vi "Argos 2.2 K1 Customized Edition.vi"(0 "PID 1 COM":refnum<visa-resource-name>="COM24", 1 "Setpoint\n START":bool, 2 "Write to File":bool, 3 "SP 1 input (°C)":dbl=10.0 min=0.0 max=1300.0, 4 "Intervall (s)":u32=1 max=600, 5 "Write/\nRead":bool=TRUE, 6 "Delay (ms)":u32=500 min=100 max=600000, 7 "Auto Tune":bool, 9 "Standby":bool, 11 "Reset\nSTOP":bool, 12 "ON":bool=TRUE caption="OFF", 13 "Get Values":bool, 15 "File Path":path) -> (8 "(°C)":dbl format="%#.3f", 14 "SP 1 is (°C)":dbl)   [LabVIEW 2013]
doc: "1. Verwendung\n\nDas Programm dient der Steuerung und Abfrage des Thermocontrollers I3252 und dem Auslesen von zwei VC 840 Messgeräten und einem Druckmessgerät Pfeiffer Single Gauge. \nDie Messgeräte werden Standardmäßig ausgelesen und erst nach Betätigung des Schalters \"Write to File\" in einer Textdatei abgespeichert. Das Eingabefeld \"Intervall\" legt den Abstand der Messpunkte fest.\nDer Setpoint für den Thermocontroller wird erst nach Betätigung des Tasters \"Setpoint START\" übernommen und angesteuert. Er wird ind den EEPROM des Gerätes geschrieben. Die Regelung kann mit Hilfe des Schalters \"Standby\" unterbrochen werden. Durch den Taster \"Reset STOPP\" kann der Setpoint aus dem EEPROM gelöscht werden.\nDie Eingabeflächen \"Constant\" und \"Thickness\" dienen der Berechnung des spezifischen Widerstands.\nDie Eingabeflächen \"User\" und \"Sample\" werden in den Header der Textdatei übernommen.\nDer Indikator \"File Path\" zeigt den aktuellen Speicherort der Textdatei an. Dieser wird nach ausschalten des Schalters \"Write to File\" gelöscht. Bei erneuten Schreiben muss ein neuer Speicherort gewählt werden. Bei Wahl desselben Speicherorts werden sämtliche bereits gespeicherte Daten gelöscht.\n\n\n2. Erläuterungen zum Blockdiagramm\n2.1 äußere Sequenz\nDie äußerte Sequenz besteht aus fünf Frames. Der erste dient der Initialisierung der Ports. Der zweite dient als Verzögerung um dem Programm genug Zeit zu geben die Ports zu öffnen. Jedoch senden die beiden VC 840 bereits Informationen an den Computer die in einem Puffer zwischengespeichert werden. Im dritten Frame wird dieser Puffer geleert. Somit kommt es zu keinem Framing Error. Desweiteren wird in diesem Frame die Startzeit der Messungen genommen. Im vierten Frame wird die eigentliche Messung und Verarbeitung der Daten durchgeführt. Die while-Schleife wird nur durch Auftreten eines Fehlers oder durch Betätigung des Stopbuttons auf dem Front Panel in der oberen linken Ecke unterbrochen. Im fünften und letzten Frame werden die Ports wieder geschlossen und beim Auftreten eines Fehlers wird das Programm automatisch gestoppt. Falls kein Fehler auftritt wird die Sequenz von vorne abgearbeitet.\n\n2.2 while-Schleife und innere Sequenz\n2.2.1 \"Event Structure\"\n2.2.1.1 Allgemein\nDer erste Frame beinhaltet ein \"Event Structure\". Dieser reagiert auf insgesamt elf verschiedene Ereignisse. Falls keines dieser Ereignisse auftreten sollte, warte die Struktur eine Millisekunde bevor die \"Event Structure\" verlassen wird. Die übrigen Ereignisse treten ein, wenn der entsprechende Kontroller eine Werteänderung erfährt.\n\n2.2.1.2 Event: Setpoint\nDieser Case besteht von außen nach innen aus einer Stacked Sequence, einer for-Loop und einer Flat Sequence die wiederum zwei \"Case Structures\" enthält. Als erstes wird bei dem Schalter \"Setpoint START\" der Blinkmodus aktiviert und bei dem Schalter \"Read Temperature\" deaktiviert. Danach folgt das eigentliche setzen des Temperatursollwerts. In der ersten Iteration wird dem Controller I3252 ein Schreibbefehl gesendet. Theoretisch kann der Setpoint in den RAM oder in den EEPROM geschrieben werden. Diese Auswahl erfolgt mit Hilfe des Schalters \"RAM\". Da das Schreiben in den RAM -Speicher aber aus diversen Gründen nicht erwünscht ist, wurde es nicht implementiert. Eine nachträgliche Implementierung ist aber leicht möglich, in dem die untere String-Konstante \"*P012\" durch \"*W012\" ersetzt wird. An diesem Befehl wird eine fünfstellige Hexadezimalzahl angehängt, die den Sollwert wiedergibt. Der Sollwert wird vorher mit zehn multipliziert, da das Komma standardmäßig nach der ersten Ziffer festgesetzt wurde (Bsp.: 800 wird gesendet um 80 einzustellen). Dieser Befehlsstrang wird an das Gerät mittels des SubVIs \"Comm_Interface\", auf welches später noch näher eingegangen wird, weitergegeben. Der durch das Gerät zurückgegebene String wird nicht verarbeitet.\nDie zweite Iteration dient dem Auslesen des eingestellten Sollwertes. Wahlweise kann der RAM- oder der EEPROM-Speicher ausgelesen werden. Die eigentliche Verarbeitung des Ausgabestrings erfolgt durch das SubVI \"Edit Setpoint\".\nDie Implementierung zur Einstellung des zweiten Setpoints erfolgt durch kopieren der ersten beiden Fälle und ersetzen der \"1\" im Befehf durch eine \"2\" (Bsp.: \"*P012\" zu \"*P022\"). Es darf aber nicht vergessen werden, dass dann ebenfalls die Anzahl der Iterationen angepasst werden muss.\nAls letztes wird der Blinkmodus des Schalters \"Setpoint START\" wieder deaktiviert.\n\n2.2.1.3 Event: Standby\nDieses Ereignis aktiviert bzw. deaktiviert als erstes den Blinckmodus des entsprechenden Schalters und sendet danach den Befehl zum aktivieren (\"*D03\") oder zum deaktivieren (\"*E03\") des Standbymodus an den Thermocontroller.\n\n2.2.1.4 Event: Set Command \nDer in das Feld \"Command shall be\" eingegebene Befehl wird an den Thermocontroller übermittlet. Die korrekte Form des Befehls ist im \"Communication Manuel\" nachzuschlagen. Das \"*\"-Zeichen wurde allerdings schon implementiert und muss somit nicht mit eingegeben werden.\n\n2.2.1.5 Event: Reset\nIn der ersten Iteration wird der Reset-Befehl an den Thermocontroller gesendet. In Folge wird der gesamte EEPROM-Speicher gelöscht. Deshalb wird in der zweiten Iteration der Setpoint aktualisiert. Dieser Befehl hat keinen Einfluss auf den RAM-Speicher. Die anschließende Wartezeit ist auf vier Sekunden festgesetzt und wurde empirisch ermittelt. Diese Zeit benötigt das Gerät um den Reset durchzuführen und für die Kommunikation wieder zur Verfügung zu stehen.\n\n2.2.1.6 Event: Auto Tune\nEs ist festgeschrieben, dass der Setpoint für die \"Auto Tune\"-Funktion wenigstens 20°C über der aktuellen Temperatur liegt. Deshalb wird zunächst der aktuelle Temperaturwert ausgelesen. Im zweiten Schritt werden zu diesem Wert zwanzig addiert und der Setpoint wird in den RAM-Speicher geschrieben. Das Schreiben in diesen Speicher ist nötig, da die \"Auto Tune\"-Funktion\" erst nach einem Reset startet. Im dritten Schritt wird der eigentliche Befehl für den \"Auto Tune\" gesendet (siehe dazu \"Communication Manuel\" S.27). Als vierte und letzte Iteration der for-Schleife folgt der bereits erwähnte Reset-Befehl. Der Temperatursollwert, der im RAM-Speicher eingetragen ist, muss zum Schluss wieder auf 0°C gesetzt werden. Die Zeit für die Ausführung des \"Auto Tune\"-Befehls wurde empirisch ermittelt und 45 s festgesetzt.\n\n2.2.1.7 Event: Write LOW/HI\nDieses Ereignis setzt die am Analogausgang anliegende Spannung fest. Normalerweise beträgt dieser Spannungswert 0-10 V. Das angeschlossene Netzteil verträgt aber maximal nur 2,3 V. Aus diesem Grund wird der \"%HIGH\" auf 23 gesetzt. Somit beträgt die maximal anliegende Spannung nur noch 23% von der maximal möglichen, d.h 2,3V. Ein niedrigerer Wert ist jederzeit möglich, genauso wie ein höherer für den Parameter \"%LOW\". Diese werden zunächst nacheinander in den RAM-Speicher geschrieben und anschließend wieder ausgelesen.\n\n2.2.1.8 Event: Set PID\nDie Werte für den PID-Regler können sowohl mit Hilfe der \"Auto Tune\"-Funktion, als auch manuell eingestellt werden. Es wird wiederum zwischen dem Schreiben in den RAM- und dem EEPROM-Speicher unterschieden. Zunächst werden die Werte für \"P\", \"I\" und \"D\", in dieser Reihenfolge, gesetzt und danach die aktuellen Werte ausgelesen.\n\n2.2.1.9 Event: Get Values\nDieses Ereignis hat zur Folge, dass die Werte für \"P\", \"I\", \"D\", \"%LOW\", \"%HIGH\" und des Setpoints wahlweise aus dem RAM- oder EEPROM-Speicher gelesen werden. Die aktuellen Werte werden nicht nur in die entsprechenden Anzeigefelder übernommen, sondern auch in die entsprechenden Eingabefelder, mit Ausnahme des Temperatursollwerts. \n\n2.2.1.10 Event: RAM\nPrinzipiell kann zwischen dem Schreiben in den RAM- oder EEPROM-Speicher des Thermocontrollers gewählt werden. Die entsprechende Schalterposition auf dem Frontpanel zeigt den aktuell verwendeten Speicher an. Die Anzeigewerte werden bei jedem Umschalten aktualisiert und sind im entsprechenden Speicher eingetragen. Die Implementierung ist identisch mit der des Ereignisses \"Get Values\". Es gilt zu beachten, dass die Werte für \"%LOW\" und \"%HIGH\" nur in den RAM-Speicher geschrieben werden können und somit auch nur aus diesem ausgelesen werden können.\n\n2.2.1.11 Event: Set Gauge to Zero\nMit Hilfe der SubVIs \"Get Pressure\" und \"Offset Display\" werden die Werte für den alten und den neuen Offset und der durch den zweiten Drucksensor ermittelt Druck ermittelt. \n\n2.2.1.12 Event: Write to File\nSollte der Schalter \"Write to File\" aktiviert werden, d.h. Schalterposition oben, so wird zunächst durch das SubVI \"Header\" ein Header für die unter \"File Path\" definierte Datei angelegt. Alle Werte, die bereits in der entsprechenden Datei stehen, werden dabei gelöscht.\n\n2.2.2 \"Timed Structures\"\nIm dritten Frame der inneren Sequenz werden die Werte für Zeitpunkt, Temperatur, Spannung, Strom und Druck ermittelt. Damit die Werte zum gleichen Zeitpunkt aufgenommen werden, werden \"Timed Sequences\" eingesetzt. Mit dem entsprechenden Schalter auf dem Front Panel unter dem Tab \"Settings\" kann gewählt werden, ob das entsprechende Gerät ausgelesen werden soll oder nicht. Die einzelnen Sequenzen werden parallel abgearbeitet, womit die Prozesszeit von diesem Frame durch der zeitintensivsten Sequenz abhängt. Dies ist in aller Regel das Auslesen der Temperatur, da ein \"Delay\" von 500 ms oder größer benötigt wird, um den Controller ordentlich ansprechen zu können.\nDie Systemzeit wird durch das SubVI \"System Time in Seconds\" in Sekunden umgerechnet und der in dem Parameter \"Starttime\" gespeicherte Wert wird abgezogen. Somit werden die Sekunden seit dem Start des Programms gezählt.\n\n2.2.3 restlichen Frames\nIm zweiten Frame wird das Intervall zwischen den einzelnen Messwerten festgelegt. Dabei wird der Wert des Parameters \"Delay\" abgezogen. Dieser Wert beträgt im Normalfall 500 ms und ist somit nicht vernachlääsigbar.\nDer Vierte Frame beinhaltet die Umrechnung des Temperatur-Strings in einen Temperaturwert durch das SubVI \"Edit Tmperature\", die Berechnung des spezifischen Widerstands durch das SubVI \"Resistivity Calculation\" und die Überprüfung des Druckwerts. Auch werden die neu gewonnen Werte in das entsprechende Shift-Register übernommen. Falls der Druckwert einen in dem Parameter \"Pressure Limit (mbar)\" festgelegten Grenzwert überschreiten sollte, wird der Thermocontroller automatisch in den Standby-Modus versetzt. Des Weiteren wird der Schalter \"Standby\" solange gesperrt, wie der Druck oberhalb des Grenzwertes liegt. Wenn der Druck wieder unter den Grenzwert gesunken ist, wird der Standby-Befehl nicht automatisch aufgehoben, sondern muss vom Benutzer durch Betätigung des entsprechenden Schalters gegeben werden.\nIm fünften Frame werden die Diagramme erstellt. Dabei wird jedes Mal von neuem das gesamte Shift-Register als Graph dargestellt. Weiterhin werden die Messwerte in ein 1D-Array geschrieben.\nDer sechste und letzte Frame beinhaltet den eigentlich Schreibvorgang der Messwerte in eine Textdatei und die Überprüfung ob ein Fehler vorliegt.\n\n2.3 SubVIs\n2.3.1 Allgemein\nDie SubVIs für die Messgeräte VC840 und das Druckmessgerät wurden aus anderen Quellen übernommen. \n\n2.3.2 \"Header\"\nIn den Header wird zunächst das aktuelle Datum und die aktuelle Zeit übernommen. Die ausgewählte Datei wird dabei überschrieben. Danach wird der Name des Benutzers und der Probe übernommen. Zum Schluss werden die Einheiten in einer Reihe, durch einen Tabulator getrennt, in den Header geschrieben.\n\n2.3.3 \"I3252 Comm Interface\"\nDieses VI stellt die Kommunikation mit dem Thermocontroller her und gibt den Ausgabe-String zurück.\n\n2.3.4 \"I3252 Edit Setpoint\"\nIm Ausgabe-String vom Thermocontroller ist an der vierten Stelle die Stelle des Dezimalpunktes verschlüsselt. Dieses Hexadezimalzahl wird herausgefiltert und an ein \"ENUM Controller\" übergeben. Dieser weist der Hexadezimalzahl eine Nummer zu, mit welcher ein Wert aus einem Array entnommen wird. Dieser Wert dient als Quotient. Der tatsächliche Wert kann somit errechnet werden.\n\n2.3.5 \"I3252 Edit Temperature\"\nDer Temperatur-String, der vom Thermocontroller zurückgegeben wird, wird in eine Dezimalzahl umgewandelt. Manchmal kommt es aus zu Dropouts, die durch dieses Programm herausgefiltert werden. Der letzte Wert wird dabei in einer \"Feedback Node\" gehalten unter der Annahme, dass sich der Temperaturwert nicht sprunghaft ändert.\n\n2.3.6 \"Resistivity Calculation\"\nDer spezifische Widerstand wird nach folgender Formel ausgerechnet. Dabei entspricht t der Dicke der Probe und C ist eine Konstante.\nrho=C*pi*t*U/(ln( 2)*I)\n\n2.3.7 \"System Time in Seconds\"\nZunächst wird die aktuelle Systemzeit ausgelesen. Danach wird diese in Stunden, Minuten und Sekunden aufgeteilt, alles in Sekunden umgerechnet und letztendlich addiert."
uses:
  <vilib>/Platform/TimedLoop/XDataNode/timing_clust.ctl
  <vilib>/Platform/TimedLoop/XDataNode/nitl_modes.ctl
  <vilib>/Platform/TimedLoop/XDataNode/wakeup.ctl
  <vilib>/Instr/_visa.llb/VISA Configure Serial Port (Instr).vi
  <vilib>/Platform/TimedLoop/scheduler/LVUserAPI/_suppVIs/Create_1kHz_TSource.vi
  <vilib>/Utility/file.llb/Write To Spreadsheet File (DBL).vi
  <vilib>/Platform/TimedLoop/XDataNode/XDataNode.xnode
  <vilib>/Platform/TimedLoop/XDataNode/XDNodeRunTimeDep.lvlib
  Argos2.0/Dependencies/Pfeiffer TPG261+262 Single+Dual Gauge/Dual Gauge.lvlib
panel:
  out "appended array":dbl[](array[numeric])
  in  "Tab Control":T1(tab)
  out "SP 2 is (°C)":dbl
  in  "SP 2 input (°C)":dbl=10.0 min=0.0 max=1300.0
  in  "Standby\n2":bool
  in  "Setpoint\n START\n2":bool
  out "Pirani (VVP1 Scroll)":cluster{dbl[], dbl[]}[](graph)
  in  "Sample":string
  in  "User":string
  out "current time (s)":dbl
  out "data logger intervall (s)":dbl
  out "loop time (s)":dbl
  in  "stop":bool
  out "CMR275 Baratron":cluster{dbl[], dbl[]}(graph)
  out "Pressure Baratron 2":dbl format="%#_4e"
  out "Pressure FullRange 2":dbl format="%#_3e"
  out "Pressure Pirani 2":dbl format="%#_3e"
  in  "Reset\nSTOP 2":bool
  out "TEMPERATURE":cluster{dbl[], dbl[]}[](graph)
  out "(°C) 2":dbl format="%#.3f"
  out "Pressure OpenPort":cluster{dbl[], dbl[]}(graph)
  out "Pressure OpenPort2":dbl caption="current"
  out "% HIGH Istwert 2":u32
  out "% LOW Istwert 2":u32
  in  "% High Sollwert 2":u32=23 max=24
  in  "% LOW Sollwert 2":u32 max=25
  in  "RAM 2":bool=TRUE caption="EEPROM"
  out "D (Rate) IstWert 2":u32
  out "I ( Reset1) Istwert 2":u32
  out "P (PB1) Istwert 2":u32 caption="actual value"
  in  "D (Rate) Sollwert 2":u32 max=3999
  in  "I ( Reset1) Sollwert 2":u32 max=3999
  in  "P (PB1) Sollwert 2":u32 caption="set value" max=9999
  in  "ON 2":bool=TRUE caption="OFF"
  in  "PID 2 COM":refnum<visa-resource-name>="COM25"
  in  "Delay (ms) 2":u32=500 min=100 max=600000
  in  "Write/\nRead \n\n2":bool=TRUE
  out "status 2":bool caption="Status"
  out "code 2":i32 caption="Code"
  out "code":i32 caption="Code"
  out "status":bool caption="Status"
  in  "Set Gauge to Zero":bool
  out "Status Gauge 1#2":i32(ring) items=["data OK", "underrange", "overrange", "sensor error", "sensor off", "no sensor", "ID error"]
  out "Pressure Gauge 1#2":dbl format="%.3e"
  out "Pressure Gauge 1#1":dbl format="%.3e"
  out "Status Gauge 1#1":i32(ring) items=["data OK", "underrange", "overrange", "sensor error", "sensor off", "no sensor", "ID error"]
  in  "TPG 1 COM":refnum<visa-resource-name>="COM23"
  in  "Pressure Limit (mbar)":dbl=1.0 min=0.0 max=1100.0
  out "Current Offset (mbar)":dbl
  in  "ON (TPG 2)":bool=TRUE caption="OFF"
  in  "ON (TPG 1)":bool=TRUE caption="OFF"
  in  "ON":bool caption="OFF"
  in  "VC 840 2":refnum<visa-resource-name>="COM8"
  out "Reading 2":dbl format="%_4f"
  out "Mode 2":enum16{"?", "Diode", "Beep", "DC", "AC"}(ring)
  out "Unit 2":string
  in  "VC 840 1":refnum<visa-resource-name>="COM1"
  out "Reading 1":dbl format="%_4f"
  out "Mode 1":enum16{"?", "Diode", "Beep", "DC", "AC"}(ring)
  out "Unit 1":string
  out "Status 1":T2
  out "Status 2":T2
  in  "ON":bool caption="OFF"
  out "% HIGH Istwert":u32
  out "% LOW Istwert":u32
  in  "% High Sollwert":u32=23 max=24
  in  "% LOW Sollwert":u32 max=25
  in  "RAM":bool=TRUE caption="EEPROM"
  out "D (Rate) IstWert":u32
  out "I ( Reset1) Istwert":u32
  out "P (PB1) Istwert":u32 caption="actual value"
  in  "D (Rate) Sollwert":u32 max=3999
  in  "I ( Reset1) Sollwert":u32 max=3999
  in  "P (PB1) Sollwert":u32 caption="set value" max=9999
  in  "Set Command":bool
  in  "Set PID":bool
  in  "Write LOW/HI":bool
  out "Command output":string
  in  "Command input":string
  in  "TPG 2 COM":refnum<visa-resource-name>="COM22"
  out "Pressure Gauge 2#2":dbl format="%.3e"
  out "Pressure Gauge 2#1":dbl format="%.3e"
  out "Status Gauge 2#2":i32(ring) items=["data OK", "underrange", "overrange", "sensor error", "sensor off", "no sensor", "ID error"]
  out "Status Gauge 2#1":i32(ring) items=["data OK", "underrange", "overrange", "sensor error", "sensor off", "no sensor", "ID error"]
  out "Command output 2":string
  in  "Command input 2":string
  in  "Set Command\n\n 2":bool
  in  "Auto Tune 2":bool
  in  "Set PID 2":bool
  in  "Write LOW/HI 2":bool
  in  "Get Values 2":bool
  out "Current":cluster{dbl[], dbl[]}(graph)
  out "Voltage":cluster{dbl[], dbl[]}(graph)
  out "Voltage (V)":dbl format="%.4e"
  out "Current (A)":dbl format="%.4e"
  out "Resistivity":cluster{dbl[], dbl[]}(graph)
  out "Resistivity (Ohm*cm)":dbl format="%.3e"
  in  "4PP constant":dbl min=0.0 max=5.0
  in  "Thickness (nm)":dbl min=0.0
  # "PID Side A"
  # "PID Side B"
  # "set \nvalue"
  # "actual \nvalue"
  # "Set \nValue\n2"
  # "Actual \nvalue 2"
  # "T (°C)"
  # "T (°C)"
  # "mbar"
  # "mbar"
  # "mbar"
  # "mbar"
  # "Pressure Measurement \n(Pfeiffer TPG261)"
  # "PID Controller (Omega Newport i3252)"
  # "PID Controller 2 (Omega Newport i3252)"
  # "P"
  # "I"
  # "D"
  # "% Low"
  # "% High"
  # "Multimeter\n#1 (VC 840)"
  # "Multimeter\n#2 (VC 840)"
  # "P"
  # "I"
  # "D"
  # "% Low"
  # "% High"
  # "Authors:  Daniel Schuster (sir-dan@web.de)\n                 Steffen Cornelius (s.cornelius@hzdr.de)\n                 Nico Spahn (x)\n\n                 premade SubVIs for readout of Pfeiffer gauge and VC840 Multimeters were used\n                 SubVI \"I3252_Comm_Interface\" is based on a modified Labview example\n\nRelease:  v1.0    \n\nVersion History:\n\nv1.1  -    28.06.2011\n             - Format des Files geändert von %.3f auf %g\n             - maximale Eingabewerte für PID begrenzt\nv1.2  -    12.07.2011\n             - Anzeige p,rho, U, V auf Scientific geändert\n             - y-Achse p,rho auf Log geändert\n             - numerische Zeitanzeige hinzugefügt\n             - 4PP Constant: pi/ln(2)=4,532 set as the default value\nv1.3  -    25.07.2011\n             - Zeitvariable auf EXT geändert, um Sprünge in Diagrammen loszuwerden\nv1.4  -   27.07.2011\n             - ALLE Variablen auf DBL zurückgesetzt wegen Formatierungsproblem im File\n             - Zeitberechnung neu gemacht (Tick count differenzen) -> Zeitsprünge korrigiert ?\n             - Delay/Intervall überarbeitet\nv1.5  -   05.12.2012\n                - Austausch der alten Pfeifer SubvIs durch neue -> nun alle 4 Kanäle des DualGauge\n                                                                                                         Controllers gleichzeitig auslesbar\n                - neue Pfeiffer SubVIs verwendet in Druckwertauslesung und Offset Berechnung des Baratron\n                  Druckes (COM5 Sensor1)\n                - Neuarragement des GUI -> FullRange und Baratron neben Temperatur auf Haupseite zu sehen\n                                                                   Pirani und OpenPort auf Meas.2 zu sehen\n                                                                   Diagnose Seite umfasst nun auch Widerstandsdiagramm\n                - Änderungen der Settingseite -> nun alle 4 Drucksensoren mit aktuellem Messwert und Gerätestatus\n                                                                           zu sehen\n                - The readout of the PID-Temperature Controller and the VC840 Multimeters was not modified\nv1.73  -  18.10.2013\n                - Layout Änderungen\nv.1.8   -  19.01.2014\n                - Änderung Layout Settings Tab\n                - Trennung der beiden TPG Dual Gauge Controls\n                -"
  # "Version 1.73    - last change 18.10.2013"
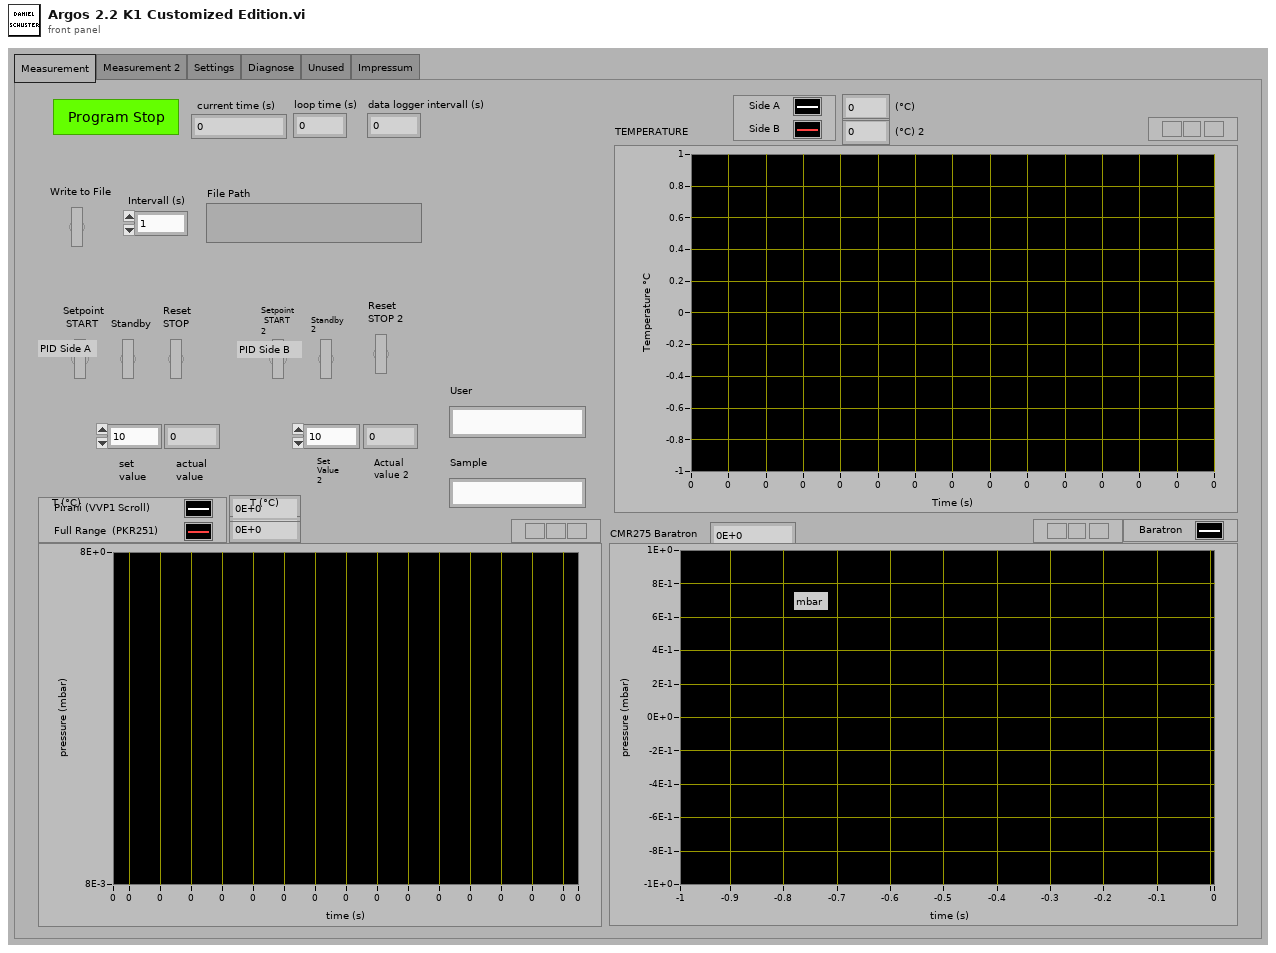
[diagram p1: front panel]
types:
  T1 = enum32{"Measurement", "Measurement 2", "Settings", "Diagnose", "Unused", "Impressum"}
  T2 = cluster{"Low Bat":bool, "Auto":bool, "Delta":bool, "Hold":bool, "RS232":bool}
  T3 = typedef "XDNodeRunTimeDep.lvlib/timing_clust.ctl" = cluster{"Expected End [f-1]":u64, "Actual End [f-1]":u64, "Finished Late? [f-1]":bool, "Expected End [i-1]":u64, "Actual End [i-1]":u64, "Finished Late? [i-1]":bool, "Expected Start [i]":u64, "Actual Start [i]":u64, "Expected Start [f]":u64, "Actual Start [f]":u64, "Source Name":string, "Structure Name":string, "Period":i64, "Deadline":i64, "Offset":i64, "Start":i64, "Priority":i32, "Timeout":i32, "Mode":T4, "Wakeup Reason":T5, "Error":errorcluster, "Source Type":string, "Secondary Source Type":string, "Global End Time":u64, "Global Start Time":u64, "Frame Duration":u64, "Iteration Duration":u64, "Assigned CPU":i32, "I/O Scan Engine Mode":u32}
  T4 = typedef "XDNodeRunTimeDep.lvlib/nitl_modes.ctl" = enum32{"No Change", "Process missed periods, maintain original phase", "Discard missed periods, maintain original phase", "Process missed periods, ignore original phase", "Discard missed periods, ignore original phase"}
  T5 = typedef "XDNodeRunTimeDep.lvlib/wakeup.ctl" = enum32{"Normal", "Aborted", "Asynchronous wakeup", "Timing source error", "Timed loop error", "Timeout"}
  T6 = enum8{"Enabled", "Disabled", "Disabled and Grayed Out"}
  T7 = cluster{"VISA resource name out":refnum<visa-resource-name>, "error out":errorcluster, "Delay (ms)":u32, "Write/\nRead":bool}
  T8 = cluster{"VISA resource name out":refnum<visa-resource-name>, "error out":errorcluster, "Delay (ms) 2":u32, "Write/\nRead \n\n2":bool}
  T9 = cluster{"TPG 2 COM":refnum<visa-resource-name>, "error out":errorcluster}
  T10 = cluster{"COM out":refnum<visa-resource-name>, "Cluster (Ausgang)":errorcluster}
  T11 = cluster{"Pressure Gauge#1":dbl, "Pressure Gauge#2":dbl}
  T12 = cluster{"TPG 1 COM":refnum<visa-resource-name>, "error out":errorcluster}
  T13 = cluster{"COM out":refnum<visa-resource-name>, "error out":errorcluster, "COM out":refnum<visa-resource-name>, "error out":errorcluster}
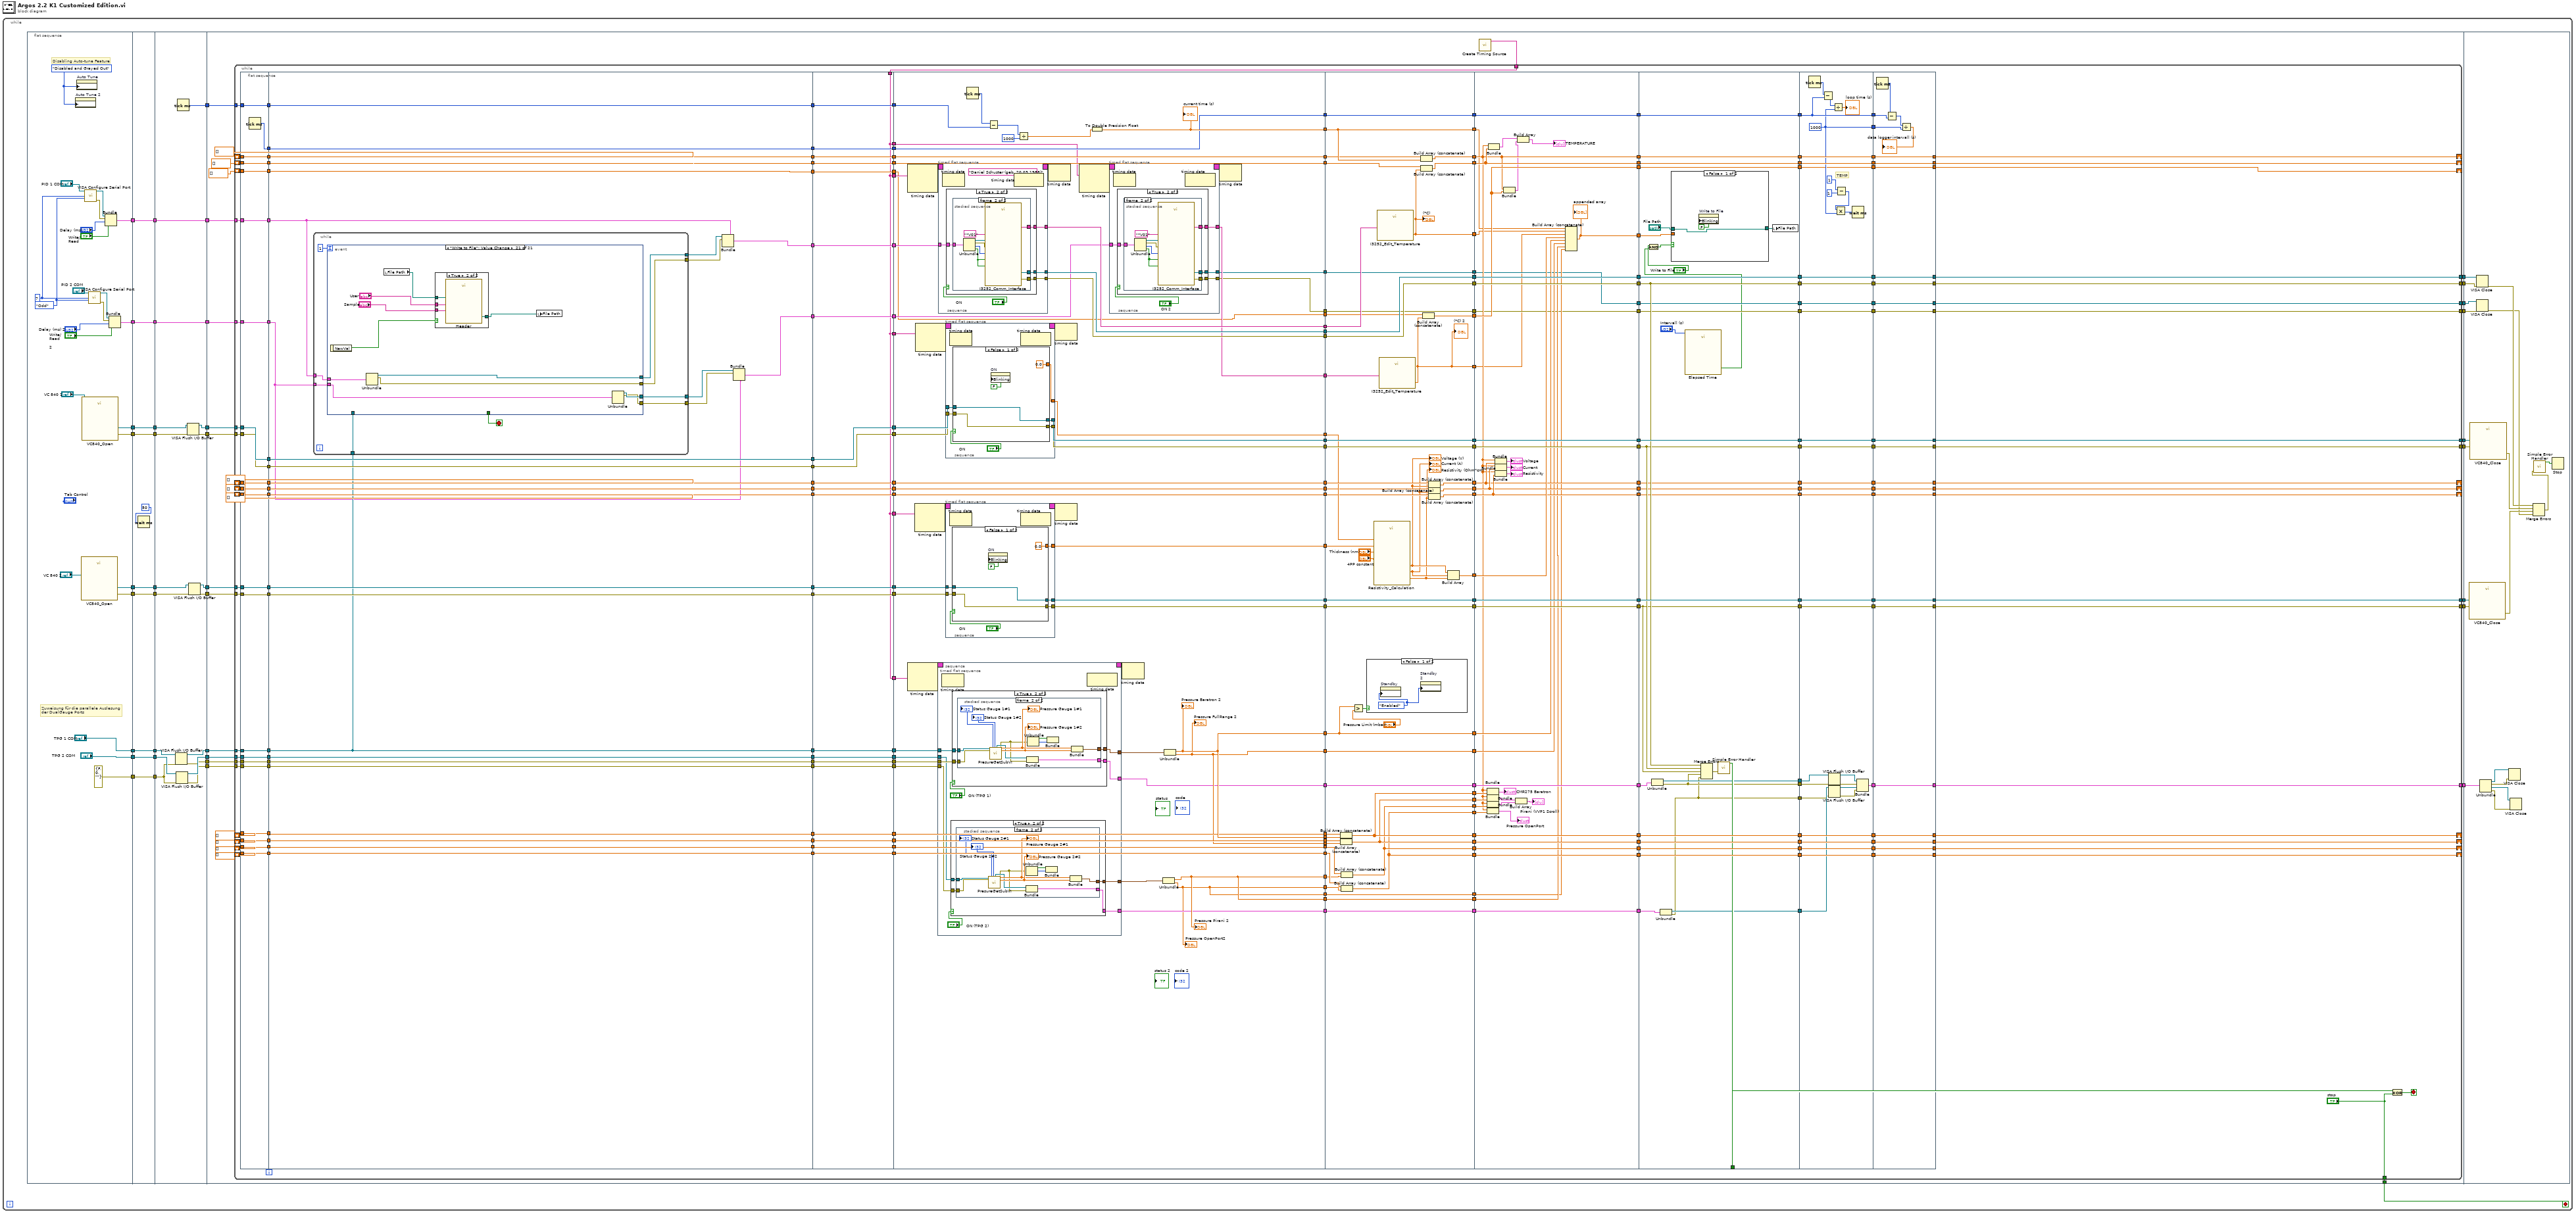
[diagram p0: block diagram]
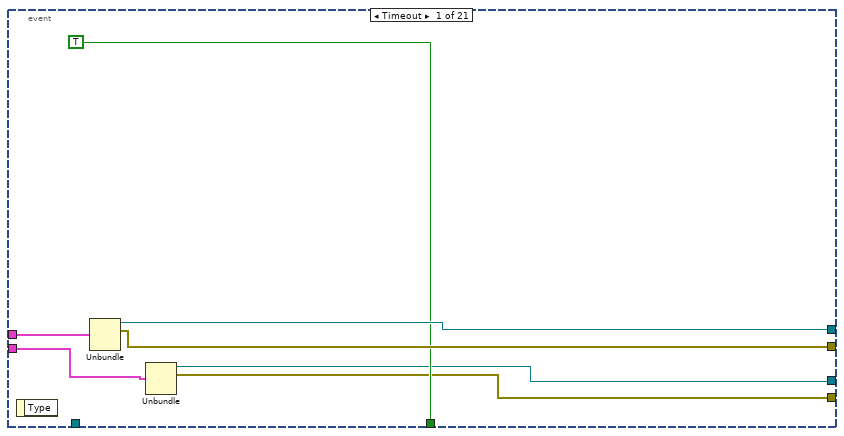
[diagram p2: hidden frame]
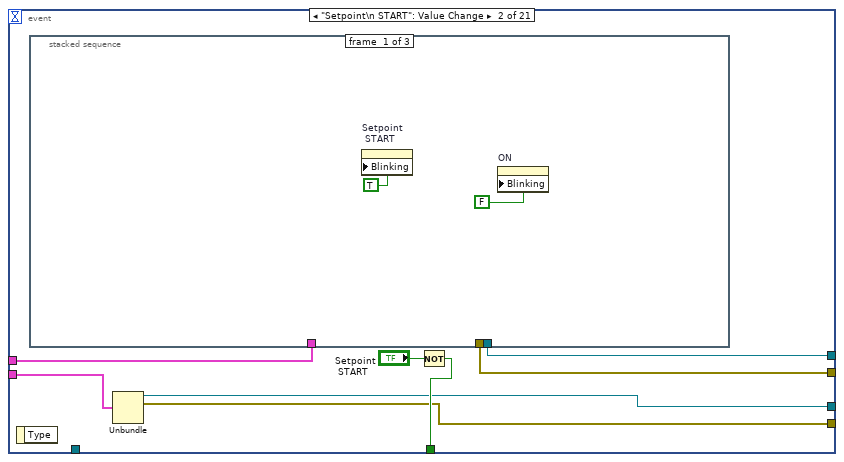
[diagram p3: hidden frame]
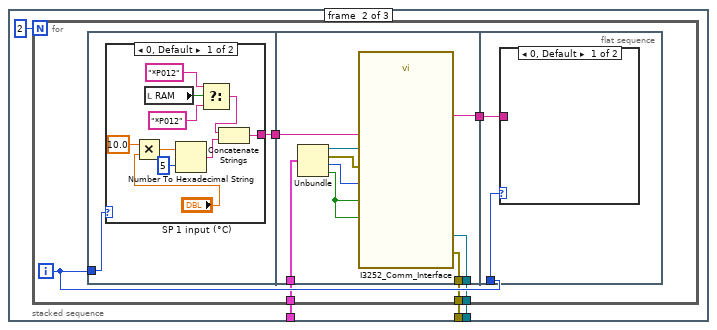
[diagram p4: hidden frame]
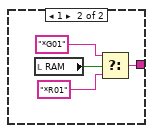
[diagram p5: hidden frame]
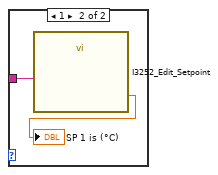
[diagram p6: hidden frame]
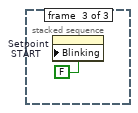
[diagram p7: hidden frame]
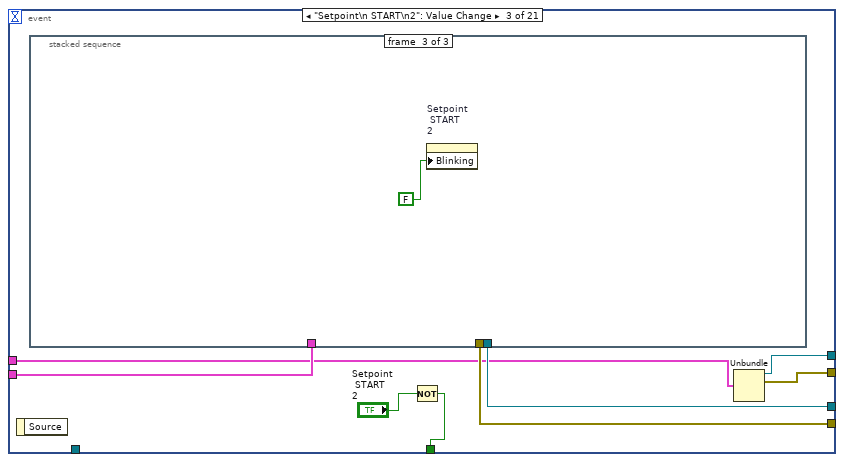
[diagram p8: hidden frame]
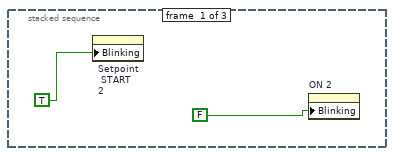
[diagram p9: hidden frame]
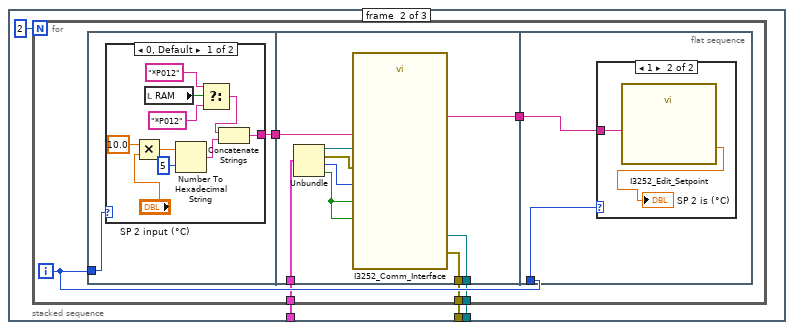
[diagram p10: hidden frame]
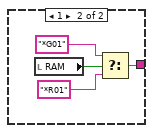
[diagram p11: hidden frame]
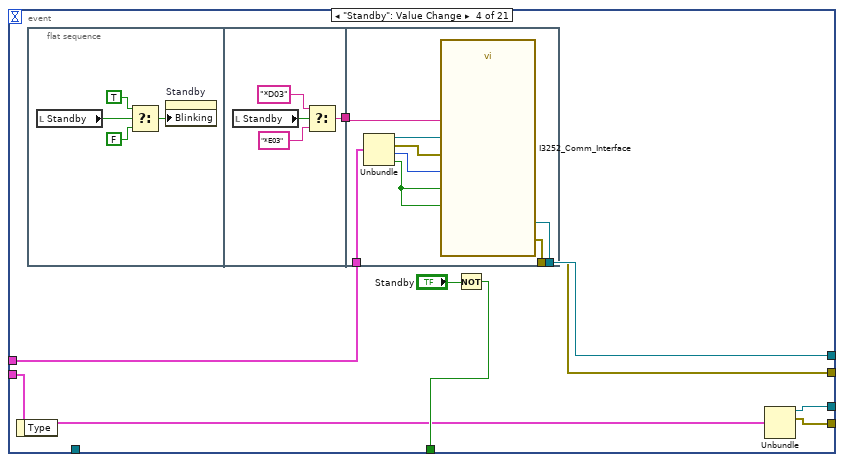
[diagram p13: hidden frame]
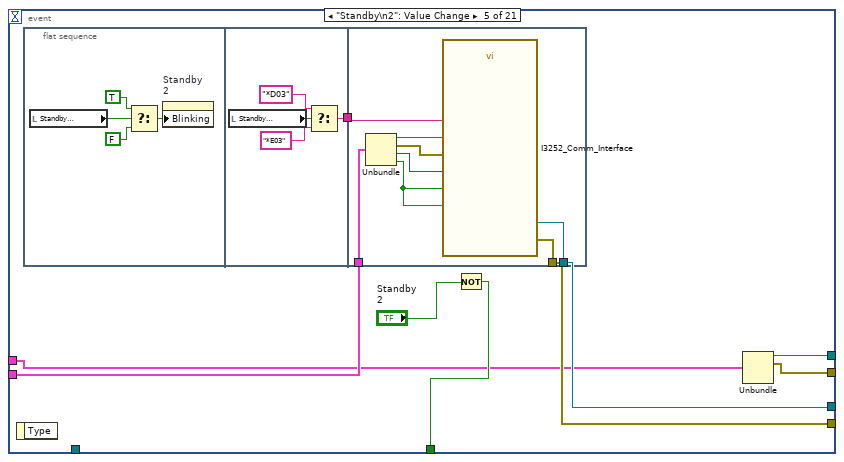
[diagram p14: hidden frame]
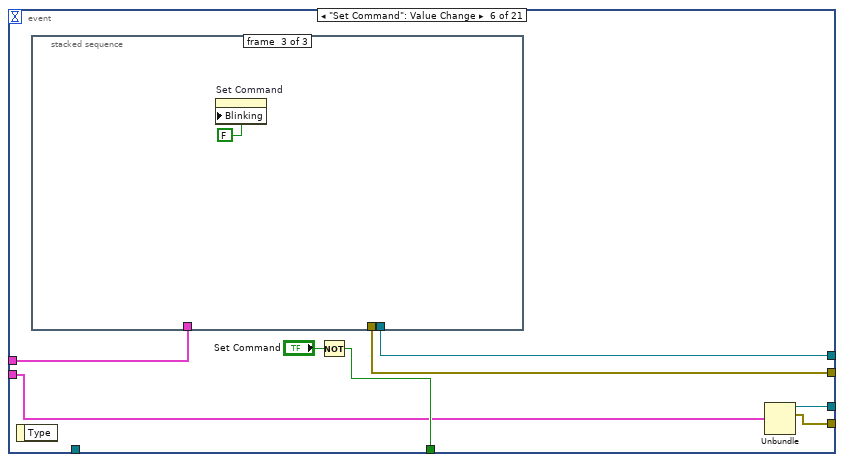
[diagram p15: hidden frame]
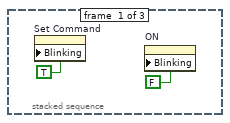
[diagram p16: hidden frame]
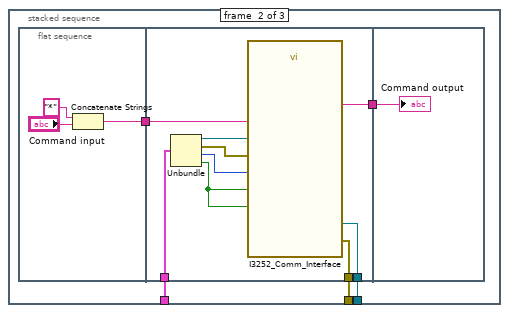
[diagram p17: hidden frame]
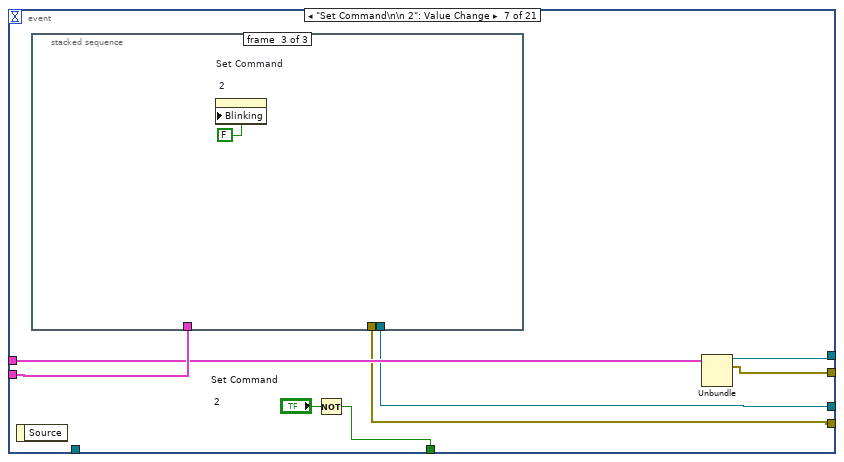
[diagram p18: hidden frame]
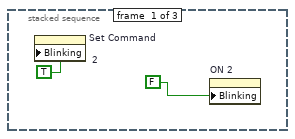
[diagram p19: hidden frame]
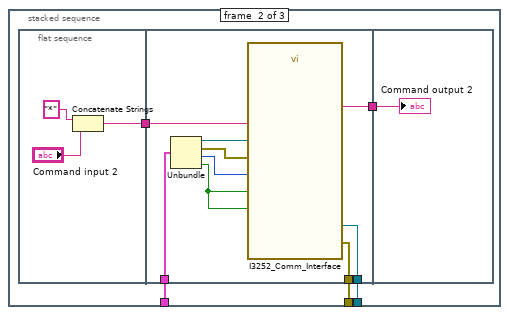
[diagram p20: hidden frame]
diagram:
  n1 = while {
    stop <- w11 stop-if-true
    n2 = flat-sequence {
      tunnel: [w62] -> w39
      tunnel: [w63] -> w38
      tunnel: [w54] -> w37
      tunnel: [w61] -> w36
      tunnel: [w60] -> w35
      tunnel: ["TPG 1 COM"] -> w34
      tunnel: ["TPG 2 COM"] -> w33
      tunnel: [errorcluster {"status"=FALSE, "code"=0, "source"=""} ("Fehler (Eingang)")] -> w8
      tunnel: [w43] -> w3
      tunnel: w39 -> [w73]
      tunnel: [w73] -> w32
      tunnel: w38 -> [w72]
      tunnel: [w72] -> w31
      tunnel: w37 -> [w71]
      tunnel: [w71] -> w30
      tunnel: w36 -> [w70]
      tunnel: [w70] -> w29
      tunnel: w35 -> [w69]
      tunnel: [w69] -> w28
      tunnel: [w67] -> w27
      tunnel: w34 -> [w67]
      tunnel: [w66] -> w26
      tunnel: w33 -> [w66]
      tunnel: [w65] -> w9
      tunnel: w8 -> [w65]
      tunnel: [w64] -> w4
      tunnel: w3 -> [w64]
      tunnel: w32 -> [w85]
      tunnel: [w84] -> w25
      tunnel: w31 -> [w86]
      tunnel: [w83] -> w24
      tunnel: w30 -> [w91]
      tunnel: [w91] -> w23
      tunnel: w29 -> [w88]
      tunnel: [w89] -> w22
      tunnel: w28 -> [w87]
      tunnel: [w90] -> w21
      tunnel: [w82] -> w20
      tunnel: [w80] -> w19
      tunnel: w27 -> [w81]
      tunnel: [w79] -> w18
      tunnel: w26 -> [w78]
      tunnel: w9 -> [w77]
      tunnel: [w76] -> w7
      tunnel: [w75] -> w6
      tunnel: [w74] -> w5
      tunnel: w4 -> [w74]
      tunnel: w25 -> [w123]
      tunnel: w24 -> [w122]
      tunnel: w23 -> [w121]
      tunnel: w22 -> [w119]
      tunnel: w21 -> [w118]
      tunnel: [w117] -> w17
      tunnel: [w116] -> w16
      tunnel: [w115] -> w15
      tunnel: [w114] -> w14
      tunnel: [w113] -> w13
      tunnel: [w112] -> w12
      tunnel: w20 -> [w106]
      tunnel: w19 -> [w105]
      tunnel: w18 -> [w104]
      tunnel: [w99] -> w11
      tunnel: [w98] -> w10
      tunnel: w7 -> [w97]
      tunnel: w6 -> [w96]
      tunnel: w5 -> [w95]
      tunnel: [w94] -> w2
      tunnel: [w93] -> w1
      tunnel: w17 -> [w1960]
      tunnel: w16 -> [w1959]
      tunnel: w15 -> [w1962]
      tunnel: w14 -> [w1961]
      tunnel: w13 -> [w1964]
      tunnel: w12 -> [w1963]
      tunnel: w10 -> [w1957]
      tunnel: w2 -> [w1952]
      tunnel: w1 -> [w1951]
      frame #0 {
        w41 = u16 7 ("data bits (8)")
        w40 = enum16{"None", "Odd", "Even", "Mark", "Space"}."Odd" ("parity (0:none)")
        w42 = T6."Disabled and Grayed Out" ("Disabled")
        # "Disabling Auto-tune Feature"
        # "Zuweisung für die parallele Auslesung\nder DualGauge Ports"
        n3 = property on="Auto Tune 2" class="Bool"("DisabledEnum"=w42) -> ()  [unwired: 2 in, 2 out]
        n4 = property on="Auto Tune" class="Bool"("DisabledEnum"=w42) -> ()  [unwired: 2 in, 2 out]
        n5 = call "VC840_Open.vi"("VISA resource name"="VC 840 2") -> ("error out"=w60:errorcluster, "VISA resource name out"=w61:refnum<visa-resource-name>)  [unwired: 1 in, 8 out]
        n6 = call "VC840_Open.vi"("VISA resource name"="VC 840 1") -> ("error out"=w63:errorcluster, "VISA resource name out"=w62:refnum<visa-resource-name>)  [unwired: 1 in, 8 out]
        n7 = call-poly "VISA Configure Serial Port"("VISA resource name"="PID 1 COM", "data bits (8)"=w41, "parity (0:none)"=w40) -> ("VISA resource name out"=w58:refnum<visa-resource-name>, "error out"=w59:errorcluster)  [unwired: 6 in, 5 out]
        n8 = call-poly "VISA Configure Serial Port"("VISA resource name"="PID 2 COM", "data bits (8)"=w41, "parity (0:none)"=w40) -> ("VISA resource name out"=w47:refnum<visa-resource-name>, "error out"=w48:errorcluster)  [unwired: 6 in, 5 out]
        n9 = Bundle("VISA resource name out"=w58, "error out"=w59, "Delay (ms)"="Delay (ms)", "Write/\nRead"="Write/\nRead") -> (w54:T7)  [unwired: 1 in]
        n10 = Bundle("VISA resource name out"=w47, "error out"=w48, "Delay (ms) 2"="Delay (ms) 2", "Write/\nRead \n\n2"="Write/\nRead \n\n2") -> (w43:T8)  [unwired: 1 in]
      }
      frame #1 {
        n11 = Wait (ms)(milliseconds to wait=u32 50) -> ()  [unwired: 1 out]
      }
      frame #2 {
        n12 = VISA Flush I/O Buffer(VISA resource name=w81, error in (no error)=w77) -> (VISA resource name out=w80:refnum<visa-resource-name>, error out=w76:errorcluster)  [unwired: 1 in]
        n13 = VISA Flush I/O Buffer(VISA resource name=w78, error in (no error)=w77) -> (VISA resource name out=w79:refnum<visa-resource-name>, error out=w75:errorcluster)  [unwired: 1 in]
        n14 = Tick Count (ms)() -> (millisecond timer value=w82:u32)
        n15 = VISA Flush I/O Buffer(VISA resource name=w85, error in (no error)=w86) -> (VISA resource name out=w84:refnum<visa-resource-name>, error out=w83:errorcluster)  [unwired: 1 in]
        n16 = VISA Flush I/O Buffer(VISA resource name=w88, error in (no error)=w87) -> (VISA resource name out=w89:refnum<visa-resource-name>, error out=w90:errorcluster)  [unwired: 1 in]
      }
      frame #3 {
        n17 = call-poly <vilib>:"Create Timing Source.vi"() -> ("name (out)"=w120:string)  [unwired: 10 in, 1 out]
        n18 = while {
          tunnel: w123 -> [w371]
          tunnel: w122 -> [w370]
          tunnel: w121 -> [w369]
          tunnel: w120 -> [w362]
          tunnel: w119 -> [w355]
          tunnel: w118 -> [w354]
          tunnel: [w350] -> w117
          tunnel: [w349] -> w116
          tunnel: [w347] -> w115
          tunnel: [w345] -> w114
          tunnel: [w343] -> w113
          tunnel: [w341] -> w112
          shift-right: [w314] -> _
          shift-left: dbl[] [] -> [w319]
          shift-right: [w292] -> _
          shift-left: dbl[] [] -> [w327]
          shift-right: [w316] -> _
          shift-left: dbl[] [] -> [w323]
          shift-right: [w289] -> _
          shift-left: dbl[] [] -> [w326]
          shift-right: [w286] -> _
          shift-left: dbl[] [] -> [w325]
          tunnel: w106 -> [w280]
          tunnel: w105 -> [w236]
          tunnel: w104 -> [w232]
          shift-right: [w190] -> _
          shift-left: dbl[] [] -> [w220]
          shift-right: [w188] -> _
          shift-left: dbl[] [] -> [w218]
          shift-right: [w186] -> _
          shift-left: dbl[] [] -> [w216]
          shift-right: [w184] -> _
          shift-left: dbl[] [] -> [w214]
          tunnel: ["stop"] -> w99
          tunnel: [w178] -> w98
          tunnel: w97 -> [w173]
          tunnel: w96 -> [w171]
          tunnel: w95 -> [w151]
          shift-right: [w143] -> _
          shift-left: dbl[] [] -> [w141]
          tunnel: [w132] -> w94
          tunnel: [w126] -> w93
          stop <- w177 stop-if-true
          n19 = flat-sequence {
            tunnel: w280 -> [w383]
            tunnel: w319 -> [w384]
            tunnel: w323 -> [w385]
            tunnel: w325 -> [w386]
            tunnel: w326 -> [w387]
            tunnel: w327 -> [w388]
            tunnel: w354 -> [w389]
            tunnel: w355 -> [w390]
            tunnel: w369 -> [w391]
            tunnel: w370 -> [w392]
            tunnel: w371 -> [w393]
            tunnel: [w393] -> w279
            tunnel: [w392] -> w278
            tunnel: [w391] -> w277
            tunnel: [w390] -> w276
            tunnel: [w389] -> w275
            tunnel: [w388] -> w274
            tunnel: [w387] -> w273
            tunnel: [w386] -> w272
            tunnel: [w385] -> w271
            tunnel: [w384] -> w270
            tunnel: [w383] -> w269
            tunnel: [w382] -> w251
            tunnel: [w381] -> w237
            tunnel: w236 -> [w381]
            tunnel: [w380] -> w233
            tunnel: w232 -> [w380]
            tunnel: [w379] -> w221
            tunnel: w220 -> [w379]
            tunnel: [w378] -> w219
            tunnel: w218 -> [w378]
            tunnel: [w377] -> w217
            tunnel: w216 -> [w377]
            tunnel: [w376] -> w215
            tunnel: w214 -> [w376]
            tunnel: [w375] -> w174
            tunnel: w173 -> [w375]
            tunnel: [w374] -> w172
            tunnel: w171 -> [w374]
            tunnel: [w373] -> w152
            tunnel: w151 -> [w373]
            tunnel: [w372] -> w142
            tunnel: w141 -> [w372]
            tunnel: [w421] -> w368
            tunnel: [w420] -> w366
            tunnel: [w416] -> w364
            tunnel: [w415] -> w359
            tunnel: [w414] -> w357
            tunnel: [w413] -> w324
            tunnel: [w412] -> w320
            tunnel: [w411] -> w300
            tunnel: [w410] -> w297
            tunnel: [w409] -> w295
            tunnel: [w408] -> w281
            tunnel: w279 -> [w421]
            tunnel: w278 -> [w420]
            tunnel: w277 -> [w419]
            tunnel: w276 -> [w415]
            tunnel: w275 -> [w414]
            tunnel: w274 -> [w411]
            tunnel: w273 -> [w410]
            tunnel: w272 -> [w409]
            tunnel: w271 -> [w413]
            tunnel: w270 -> [w412]
            tunnel: w269 -> [w408]
            tunnel: [w407] -> w252
            tunnel: w251 -> [w407]
            tunnel: w237 -> [w405]
            tunnel: [w405] -> w234
            tunnel: w233 -> [w406]
            tunnel: [w406] -> w230
            tunnel: w221 -> [w404]
            tunnel: w219 -> [w403]
            tunnel: w217 -> [w402]
            tunnel: w215 -> [w401]
            tunnel: [w404] -> w213
            tunnel: [w403] -> w209
            tunnel: [w402] -> w206
            tunnel: [w401] -> w205
            tunnel: w174 -> [w400]
            tunnel: w172 -> [w399]
            tunnel: [w400] -> w169
            tunnel: [w399] -> w167
            tunnel: w152 -> [w395]
            tunnel: [w394] -> w149
            tunnel: w142 -> [w398]
            tunnel: [w398] -> w140
            tunnel: w368 -> [w1472]
            tunnel: [w1472] -> w367
            tunnel: w366 -> [w1471]
            tunnel: [w1471] -> w365
            tunnel: w364 -> [w1468]
            tunnel: [w1468] -> w363
            tunnel: w362 -> [w1450]
            tunnel: [w1450] -> w361
            tunnel: [w1450] -> w360
            tunnel: w359 -> [w1470]
            tunnel: [w1470] -> w358
            tunnel: w357 -> [w1469]
            tunnel: [w1469] -> w356
            tunnel: [w1450] -> w353
            tunnel: [w1450] -> w339
            tunnel: w324 -> [w1467]
            tunnel: [w1467] -> w322
            tunnel: w320 -> [w1466]
            tunnel: [w1466] -> w317
            tunnel: [w1465] -> w301
            tunnel: w300 -> [w1465]
            tunnel: [w1464] -> w298
            tunnel: w297 -> [w1464]
            tunnel: [w1463] -> w296
            tunnel: w295 -> [w1463]
            tunnel: [w1462] -> w282
            tunnel: w281 -> [w1462]
            tunnel: [w1461] -> w253
            tunnel: w252 -> [w1461]
            tunnel: [w1460] -> w235
            tunnel: w234 -> [w1460]
            tunnel: [w1459] -> w231
            tunnel: w230 -> [w1459]
            tunnel: w213 -> [w1458]
            tunnel: [w1458] -> w212
            tunnel: [w1457] -> w210
            tunnel: w209 -> [w1457]
            tunnel: [w1456] -> w208
            tunnel: w206 -> [w1456]
            tunnel: w205 -> [w1455]
            tunnel: [w1455] -> w204
            tunnel: [w1454] -> w170
            tunnel: w169 -> [w1454]
            tunnel: [w1453] -> w168
            tunnel: w167 -> [w1453]
            tunnel: [w1452] -> w150
            tunnel: w149 -> [w1452]
            tunnel: w140 -> [w1451]
            tunnel: [w1451] -> w139
            tunnel: [w1450] -> w125
            tunnel: [w1503] -> w338
            tunnel: w367 -> [w1532]
            tunnel: w365 -> [w1531]
            tunnel: w363 -> [w1528]
            tunnel: w361 -> [w1527]
            tunnel: w360 -> [w1526]
            tunnel: w358 -> [w1516]
            tunnel: w356 -> [w1515]
            tunnel: w353 -> [w1517]
            tunnel: [w1513] -> w337
            tunnel: [w1514] -> w336
            tunnel: [w1525] -> w335
            tunnel: [w1524] -> w334
            tunnel: [w1523] -> w333
            tunnel: [w1522] -> w332
            tunnel: w339 -> [w1512]
            tunnel: [w1511] -> w331
            tunnel: [w1510] -> w330
            tunnel: [w1494] -> w329
            tunnel: [w1509] -> w328
            tunnel: w322 -> [w1508]
            tunnel: [w1508] -> w321
            tunnel: [w1507] -> w318
            tunnel: w317 -> [w1507]
            tunnel: w301 -> [w1506]
            tunnel: [w1506] -> w299
            tunnel: w298 -> [w1505]
            tunnel: w296 -> [w1504]
            tunnel: [w1505] -> w294
            tunnel: [w1504] -> w293
            tunnel: w282 -> [w1502]
            tunnel: [w1498] -> w254
            tunnel: w253 -> [w1498]
            tunnel: w235 -> [w1496]
            tunnel: w231 -> [w1495]
            tunnel: [w1489] -> w229
            tunnel: [w1494] -> w228
            tunnel: [w1492] -> w227
            tunnel: [w1490] -> w226
            tunnel: w212 -> [w1493]
            tunnel: [w1493] -> w211
            tunnel: w210 -> [w1492]
            tunnel: w208 -> [w1491]
            tunnel: [w1491] -> w207
            tunnel: w204 -> [w1490]
            tunnel: [w1489] -> w182
            tunnel: [w1488] -> w179
            tunnel: w170 -> [w1487]
            tunnel: w168 -> [w1486]
            tunnel: [w1483] -> w163
            tunnel: [w1481] -> w162
            tunnel: [w1483] -> w161
            tunnel: [w1482] -> w157
            tunnel: [w1481] -> w154
            tunnel: w150 -> [w1478]
            tunnel: [w1477] -> w148
            tunnel: w139 -> [w1476]
            tunnel: [w1476] -> w138
            tunnel: [w1475] -> w136
            tunnel: [w1474] -> w127
            tunnel: w125 -> [w1473]
            tunnel: w338 -> [w1779]
            tunnel: [w1776] -> w312
            tunnel: w337 -> [w1792]
            tunnel: [w1792] -> w311
            tunnel: w336 -> [w1791]
            tunnel: [w1791] -> w310
            tunnel: w335 -> [w1790]
            tunnel: [w1790] -> w309
            tunnel: w334 -> [w1789]
            tunnel: [w1789] -> w308
            tunnel: w333 -> [w1788]
            tunnel: [w1788] -> w307
            tunnel: w332 -> [w1787]
            tunnel: [w1787] -> w306
            tunnel: [w1780] -> w305
            tunnel: w331 -> [w1773]
            tunnel: w330 -> [w1781]
            tunnel: w329 -> [w1780]
            tunnel: w328 -> [w1782]
            tunnel: [w1779] -> w304
            tunnel: w321 -> [w1778]
            tunnel: w318 -> [w1777]
            tunnel: [w1775] -> w303
            tunnel: [w1763] -> w302
            tunnel: w299 -> [w1774]
            tunnel: w294 -> [w1771]
            tunnel: w293 -> [w1770]
            tunnel: [w1772] -> w290
            tunnel: [w1769] -> w287
            tunnel: [w1768] -> w284
            tunnel: [w1764] -> w283
            tunnel: [w1762] -> w255
            tunnel: w254 -> [w1762]
            tunnel: w229 -> [w1761]
            tunnel: w228 -> [w1760]
            tunnel: w227 -> [w1759]
            tunnel: w226 -> [w1757]
            tunnel: [w1755] -> w225
            tunnel: [w1754] -> w224
            tunnel: [w1753] -> w223
            tunnel: [w1752] -> w222
            tunnel: w211 -> [w1756]
            tunnel: w207 -> [w1758]
            tunnel: [w1755] -> w203
            tunnel: [w1754] -> w202
            tunnel: [w1753] -> w201
            tunnel: [w1752] -> w200
            tunnel: [w1751] -> w183
            tunnel: w182 -> [w1751]
            tunnel: [w1750] -> w180
            tunnel: w179 -> [w1750]
            tunnel: w163 -> [w1749]
            tunnel: w162 -> [w1748]
            tunnel: w161 -> [w1747]
            tunnel: [w1747] -> w160
            tunnel: [w1746] -> w158
            tunnel: w157 -> [w1746]
            tunnel: w154 -> [w1745]
            tunnel: [w1745] -> w153
            tunnel: w148 -> [w1744]
            tunnel: [w1743] -> w147
            tunnel: w138 -> [w1742]
            tunnel: [w1741] -> w137
            tunnel: w136 -> [w1741]
            tunnel: [w1740] -> w128
            tunnel: w127 -> [w1740]
            tunnel: [w1739] -> w124
            tunnel: w312 -> [w1797]
            tunnel: [w1840] -> w352
            tunnel: [w1839] -> w351
            tunnel: w311 -> [w1839]
            tunnel: [w1834] -> w348
            tunnel: w310 -> [w1834]
            tunnel: [w1838] -> w346
            tunnel: w309 -> [w1838]
            tunnel: [w1837] -> w344
            tunnel: w308 -> [w1837]
            tunnel: [w1836] -> w342
            tunnel: w307 -> [w1836]
            tunnel: [w1835] -> w340
            tunnel: w306 -> [w1835]
            tunnel: w305 -> [w1825]
            tunnel: w304 -> [w1798]
            tunnel: w303 -> [w1807]
            tunnel: [w1807] -> w315
            tunnel: w302 -> [w1826]
            tunnel: [w1826] -> w313
            tunnel: [w1827] -> w291
            tunnel: w290 -> [w1827]
            tunnel: [w1828] -> w288
            tunnel: w287 -> [w1828]
            tunnel: [w1829] -> w285
            tunnel: w284 -> [w1829]
            tunnel: w283 -> [w1833]
            tunnel: [w1824] -> w256
            tunnel: w255 -> [w1824]
            tunnel: w225 -> [w1822]
            tunnel: w224 -> [w1821]
            tunnel: w223 -> [w1820]
            tunnel: w222 -> [w1819]
            tunnel: w203 -> [w1818]
            tunnel: w202 -> [w1817]
            tunnel: w201 -> [w1816]
            tunnel: w200 -> [w1815]
            tunnel: [w1818] -> w198
            tunnel: [w1817] -> w196
            tunnel: [w1816] -> w194
            tunnel: [w1815] -> w192
            tunnel: w183 -> [w1814]
            tunnel: [w1813] -> w181
            tunnel: w180 -> [w1813]
            tunnel: w160 -> [w1811]
            tunnel: [w1810] -> w159
            tunnel: w158 -> [w1810]
            tunnel: w153 -> [w1809]
            tunnel: w147 -> [w1808]
            tunnel: [w1808] -> w144
            tunnel: w137 -> [w1806]
            tunnel: [w1806] -> w133
            tunnel: [w1805] -> w129
            tunnel: w128 -> [w1805]
            tunnel: w124 -> [w1796]
            tunnel: w352 -> [w1860]
            tunnel: w351 -> [w1874]
            tunnel: w348 -> [w1868]
            tunnel: w346 -> [w1873]
            tunnel: w344 -> [w1870]
            tunnel: w342 -> [w1872]
            tunnel: w340 -> [w1871]
            tunnel: w315 -> [w1865]
            tunnel: w313 -> [w1864]
            tunnel: w291 -> [w1863]
            tunnel: w288 -> [w1862]
            tunnel: w285 -> [w1861]
            tunnel: [w1854] -> w176
            tunnel: [w1874] -> w268
            tunnel: [w1868] -> w267
            tunnel: [w1873] -> w266
            tunnel: [w1870] -> w265
            tunnel: [w1872] -> w264
            tunnel: [w1871] -> w263
            tunnel: [w1865] -> w262
            tunnel: [w1864] -> w261
            tunnel: [w1863] -> w260
            tunnel: [w1862] -> w259
            tunnel: [w1861] -> w258
            tunnel: [w1859] -> w257
            tunnel: w256 -> [w1859]
            tunnel: [w1858] -> w199
            tunnel: w198 -> [w1858]
            tunnel: [w1857] -> w197
            tunnel: w196 -> [w1857]
            tunnel: [w1856] -> w195
            tunnel: w194 -> [w1856]
            tunnel: [w1855] -> w193
            tunnel: w192 -> [w1855]
            tunnel: w181 -> [w1853]
            tunnel: [w1852] -> w166
            tunnel: [w1851] -> w165
            tunnel: w159 -> [w1850]
            tunnel: [w1849] -> w156
            tunnel: [w1848] -> w155
            tunnel: [w1847] -> w145
            tunnel: w144 -> [w1847]
            tunnel: [w1846] -> w134
            tunnel: w133 -> [w1846]
            tunnel: [w1845] -> w130
            tunnel: w129 -> [w1845]
            tunnel: w268 -> [w1925]
            tunnel: w267 -> [w1924]
            tunnel: w266 -> [w1923]
            tunnel: w265 -> [w1922]
            tunnel: w264 -> [w1921]
            tunnel: w263 -> [w1920]
            tunnel: w262 -> [w1919]
            tunnel: w261 -> [w1918]
            tunnel: w260 -> [w1917]
            tunnel: w259 -> [w1916]
            tunnel: w258 -> [w1915]
            tunnel: w257 -> [w1909]
            tunnel: [w1925] -> w250
            tunnel: [w1924] -> w249
            tunnel: [w1923] -> w248
            tunnel: [w1922] -> w247
            tunnel: [w1921] -> w246
            tunnel: [w1920] -> w245
            tunnel: [w1919] -> w244
            tunnel: [w1918] -> w243
            tunnel: [w1917] -> w242
            tunnel: [w1916] -> w241
            tunnel: [w1915] -> w240
            tunnel: [w1909] -> w239
            tunnel: [w1908] -> w238
            tunnel: w199 -> [w1906]
            tunnel: w197 -> [w1905]
            tunnel: w195 -> [w1904]
            tunnel: w193 -> [w1903]
            tunnel: [w1906] -> w191
            tunnel: [w1905] -> w189
            tunnel: [w1904] -> w187
            tunnel: [w1903] -> w185
            tunnel: w166 -> [w1902]
            tunnel: w165 -> [w1901]
            tunnel: [w1896] -> w164
            tunnel: w156 -> [w1895]
            tunnel: w155 -> [w1894]
            tunnel: [w1893] -> w146
            tunnel: w145 -> [w1893]
            tunnel: [w1892] -> w135
            tunnel: w134 -> [w1892]
            tunnel: [w1891] -> w131
            tunnel: w130 -> [w1891]
            tunnel: [w1939] -> w286
            tunnel: [w1940] -> w289
            tunnel: [w1941] -> w292
            tunnel: [w1942] -> w314
            tunnel: [w1943] -> w316
            tunnel: [w1944] -> w341
            tunnel: [w1945] -> w343
            tunnel: [w1946] -> w345
            tunnel: [w1947] -> w347
            tunnel: [w1948] -> w349
            tunnel: [w1949] -> w350
            tunnel: w250 -> [w1949]
            tunnel: w249 -> [w1948]
            tunnel: w248 -> [w1947]
            tunnel: w247 -> [w1946]
            tunnel: w246 -> [w1945]
            tunnel: w245 -> [w1944]
            tunnel: w244 -> [w1943]
            tunnel: w243 -> [w1942]
            tunnel: w242 -> [w1941]
            tunnel: w241 -> [w1940]
            tunnel: w240 -> [w1939]
            tunnel: w239 -> [w1935]
            tunnel: w238 -> [w1934]
            tunnel: [w1933] -> w190
            tunnel: w191 -> [w1933]
            tunnel: [w1932] -> w188
            tunnel: w189 -> [w1932]
            tunnel: [w1931] -> w186
            tunnel: w187 -> [w1931]
            tunnel: [w1930] -> w184
            tunnel: w185 -> [w1930]
            tunnel: [w1929] -> w178
            tunnel: w164 -> [w1929]
            tunnel: [w1928] -> w143
            tunnel: w146 -> [w1928]
            tunnel: w135 -> [w1927]
            tunnel: [w1927] -> w132
            tunnel: w131 -> [w1926]
            tunnel: [w1926] -> w126
            frame #0 {
              n20 = Tick Count (ms)() -> (millisecond timer value=w382:u32)
            }
            frame #1 {
              n21 = while {
                tunnel: w419 -> [w429]
                tunnel: [w428] -> w418
                tunnel: [w424] -> w417
                tunnel: w405 -> [w426]
                tunnel: w395 -> [w425]
                tunnel: [w423] -> w397
                tunnel: [w422] -> w396
                stop <- w430 stop-if-true
                n22 = event shown="[20] \"Write to File\": Value Change" {
                  selector: _ -> [_ _ _ _ _ _ _ _ _ _ _ _ _ _ _ _ _ _ _ _ _]
                  dyn-events: _ -> [_ _ _ _ _ _ _ _ _ _ _ _ _ _ _ _ _ _ _ _ _]
                  timeout: 1 -> [_ _ _ _ _ _ _ _ _ _ _ _ _ _ _ _ _ _ _ _ _]
                  tunnel: [TRUE ("Set Gauge to Zero") w444 w495 w546 w571 w595 w624 w653 w692 w730 w788 w847 w901 w955 w1037 w1119 w1193 w1267 w1341 "Set Gauge to Zero" _] -> w430
                  tunnel: w429 -> [w437 w443 w490 w543 w565 w593 w621 w649 w687 w729 w783 w843 w899 w953 w1035 w1117 w1189 w1265 w1339 w1419 w1444]
                  tunnel: [w436 w442 w489 w542 w564 w592 w618 w651 w686 w727 w785 w845 w898 w952 w1034 w1116 w1191 w1264 w1338 w1418 w1443] -> w428
                  tunnel: [w435 w441 w488 w541 w563 w591 w617 w650 w685 w728 w784 w844 w897 w951 w1033 w1115 w1190 w1263 w1337 w1417 w1442] -> w424
                  tunnel: w426 -> [_ _ _ _ _ _ _ _ _ _ _ _ _ _ _ _ _ _ _ w1415 _]
                  tunnel: w425 -> [w433 w440 w493 w540 w568 w590 w622 w646 w690 w726 w782 w842 w896 w950 w1030 w1114 w1188 w1262 w1336 w1410 w1436]
                  tunnel: [w431 w439 w492 w539 w567 w589 w620 w648 w689 w725 w787 w841 w895 w949 w1032 w1113 w1187 w1261 w1335 w1409 w1435] -> w423
                  tunnel: [w432 w438 w491 w538 w566 w588 w619 w647 w688 w724 w786 w840 w894 w948 w1031 w1112 w1186 w1260 w1334 w1408 w1434] -> w422
                  event Timeout {
                    n23 = event-data() -> ()  [unwired: 1 in, 1 out]
                    n24 = Unbundle(w437) -> ("VISA resource name out"=w436:refnum<visa-resource-name>, "error out"=w435:errorcluster)  [unwired: 2 out]
                    n25 = Unbundle(w433) -> ("VISA resource name out"=w431:refnum<visa-resource-name>, "error out"=w432:errorcluster)  [unwired: 2 out]
                  }
                  event "Setpoint\n START": Value Change {
                    n26 = event-data() -> ()  [unwired: 1 in, 1 out]
                    n27 = stacked-sequence {
                      tunnel: w443 -> [_ w450 _]
                      tunnel: [_ w449 _] -> w441
                      tunnel: [_ w448 _] -> w442
                      frame #0 {
                        n28 = property on="Setpoint\n START" class="Bool"("Blinking"=TRUE) -> ()  [unwired: 2 in, 2 out]
                        n29 = property on="ON" class="Bool (strict)"("Blinking"=FALSE) -> ()  [unwired: 2 in, 2 out]
                      }
                      frame #1 {
                        n30 = for {
                          N: 2 -> [_]
                          tunnel: w450 -> [w454]
                          tunnel: [w453] -> w449
                          tunnel: [w452] -> w448
                          i -> [w456]
                          n31 = flat-sequence {
                            tunnel: [w459] -> w455
                            tunnel: w456 -> [w458]
                            tunnel: [w477] -> w457
                            tunnel: w455 -> [w476]
                            tunnel: w454 -> [w478]
                            tunnel: [w475] -> w453
                            tunnel: [w474] -> w452
                            tunnel: w457 -> [w484]
                            tunnel: w456 -> [w483]
                            frame #0 {
                              n32 = case shown="0, Default" w458 {
                                tunnel: [w468 w470] -> w459
                                frame 0, Default {
                                n33 = Multiply(x=10.0, y="SP 1 input (°C)") -> (x*y=w465:dbl)
                                n34 = local read "RAM"() -> (w463:bool)
                                n35 = Number To Hexadecimal String(1:i16 5 ("width (-)"), 2:w465) -> (0:w467:string)
                                n36 = Select(t="*P012", s=w463, f="*P012") -> (s? t:f=w460:string)
                                n37 = Concatenate Strings(w460, w467) -> (w468:string)
                                }
                                frame 1 {
                                n38 = local read "RAM"() -> (w473:bool)
                                n39 = Select(t="*G01", s=w473, f="*R01") -> (s? t:f=w470:string)
                                }
                              }
                            }
                            frame #1 {
                              n40 = Unbundle(w478) -> ("VISA resource name out"=w479:refnum<visa-resource-name>, "error out"=w481:errorcluster, "Delay (ms)"=w480:u32, "Write/\nRead"=w482:bool)
                              n41 = call "I3252_Comm_Interface.vi"("VISA resource name in"=w479, "error in"=w481, "Delay (ms)"=w480, "Write"=w482, "String to Write"=w476, "Read"=w482) -> ("VISA resource name out"=w474:refnum<visa-resource-name>, "error out"=w475:errorcluster, "Read String"=w477:string)  [unwired: 2 in]
                            }
                            frame #2 {
                              n42 = case shown="0, Default" w483 {
                                tunnel: w484 -> [_ w486]
                                frame 0, Default {
                                }
                                frame 1 {
                                n43 = call "I3252_Edit_Setpoint.vi"("Read String"=w486) -> ("Setpoint is"=→"SP 1 is (°C)":dbl)
                                }
                              }
                            }
                          }
                        }
                      }
                      frame #2 {
                        n44 = property on="Setpoint\n START" class="Bool"("Blinking"=FALSE) -> ()  [unwired: 2 in, 2 out]
                      }
                    }
                    n45 = Unbundle(w440) -> ("VISA resource name out"=w439:refnum<visa-resource-name>, "error out"=w438:errorcluster)  [unwired: 2 out]
                    n46 = Not(x="Setpoint\n START") -> (.not. x?=w444:bool)
                  }
                  event "Setpoint\n START\n2": Value Change {
                    n47 = event-data() -> ()  [unwired: 1 in, 1 out]
                    n48 = stacked-sequence {
                      tunnel: w493 -> [_ w500 _]
                      tunnel: [_ w499 _] -> w491
                      tunnel: [_ w498 _] -> w492
                      frame #0 {
                        n49 = property on="Setpoint\n START\n2" class="Bool"("Blinking"=TRUE) -> ()  [unwired: 2 in, 2 out]
                        n50 = property on="ON 2" class="Bool (strict)"("Blinking"=FALSE) -> ()  [unwired: 2 in, 2 out]
                      }
                      frame #1 {
                        n51 = for {
                          N: 2 -> [_]
                          tunnel: w500 -> [w504]
                          tunnel: [w503] -> w499
                          tunnel: [w502] -> w498
                          i -> [w506]
                          n52 = flat-sequence {
                            tunnel: [w509] -> w505
                            tunnel: w506 -> [w508]
                            tunnel: [w527] -> w507
                            tunnel: w505 -> [w526]
                            tunnel: w504 -> [w528]
                            tunnel: [w525] -> w503
                            tunnel: [w524] -> w502
                            tunnel: w507 -> [w534]
                            tunnel: w506 -> [w533]
                            frame #0 {
                              n53 = case shown="0, Default" w508 {
                                tunnel: [w518 w520] -> w509
                                frame 0, Default {
                                n54 = Multiply(x=10.0, y="SP 2 input (°C)") -> (x*y=w516:dbl)
                                n55 = local read "RAM"() -> (w514:bool)
                                n56 = Number To Hexadecimal String(1:i16 5 ("width (-)"), 2:w516) -> (0:w517:string)
                                n57 = Select(t="*P012", s=w514, f="*P012") -> (s? t:f=w511:string)
                                n58 = Concatenate Strings(w511, w517) -> (w518:string)
                                }
                                frame 1 {
                                n59 = local read "RAM"() -> (w523:bool)
                                n60 = Select(t="*G01", s=w523, f="*R01") -> (s? t:f=w520:string)
                                }
                              }
                            }
                            frame #1 {
                              n61 = Unbundle(w528) -> ("VISA resource name out"=w529:refnum<visa-resource-name>, "error out"=w531:errorcluster, "Delay (ms) 2"=w530:u32, "Write/\nRead \n\n2"=w532:bool)
                              n62 = call "I3252_Comm_Interface.vi"("VISA resource name in"=w529, "error in"=w531, "Delay (ms)"=w530, "Write"=w532, "String to Write"=w526, "Read"=w532) -> ("VISA resource name out"=w524:refnum<visa-resource-name>, "error out"=w525:errorcluster, "Read String"=w527:string)  [unwired: 2 in]
                            }
                            frame #2 {
                              n63 = case shown="1" w533 {
                                tunnel: w534 -> [_ w536]
                                frame 0, Default {
                                }
                                frame 1 {
                                n64 = call "I3252_Edit_Setpoint.vi"("Read String"=w536) -> ("Setpoint is"=→"SP 2 is (°C)":dbl)
                                }
                              }
                            }
                          }
                        }
                      }
                      frame #2 {
                        n65 = property on="Setpoint\n START\n2" class="Bool"("Blinking"=FALSE) -> ()  [unwired: 2 in, 2 out]
                      }
                    }
                    n66 = Not(x="Setpoint\n START\n2") -> (.not. x?=w495:bool)
                    n67 = Unbundle(w490) -> ("VISA resource name out"=w489:refnum<visa-resource-name>, "error out"=w488:errorcluster)  [unwired: 2 out]
                  }
                  event "Standby": Value Change {
                    n68 = event-data() -> ()  [unwired: 1 in, 1 out]
                    n69 = flat-sequence {
                      tunnel: [w554] -> w544
                      tunnel: w544 -> [w558]
                      tunnel: w543 -> [w557]
                      tunnel: [w556] -> w541
                      tunnel: [w555] -> w542
                      frame #0 {
                        n70 = local read "Standby"() -> (w547:bool)
                        n71 = Select(t=TRUE, s=w547, f=FALSE) -> (s? t:f=w550:bool)
                        n72 = property on="Standby" class="Bool (strict)"("Blinking"=w550) -> ()  [unwired: 2 in, 2 out]
                      }
                      frame #1 {
                        n73 = local read "Standby"() -> (w552:bool)
                        n74 = Select(t="*D03", s=w552, f="*E03") -> (s? t:f=w554:string)
                      }
                      frame #2 {
                        n75 = Unbundle(w557) -> ("VISA resource name out"=w559:refnum<visa-resource-name>, "error out"=w561:errorcluster, "Delay (ms)"=w560:u32, "Write/\nRead"=w562:bool)
                        n76 = call "I3252_Comm_Interface.vi"("VISA resource name in"=w559, "error in"=w561, "Delay (ms)"=w560, "Write"=w562, "String to Write"=w558, "Read"=w562) -> ("VISA resource name out"=w555:refnum<visa-resource-name>, "error out"=w556:errorcluster)  [unwired: 2 in, 1 out]
                      }
                    }
                    n77 = Not(x="Standby") -> (.not. x?=w546:bool)
                    n78 = Unbundle(w540) -> ("VISA resource name out"=w539:refnum<visa-resource-name>, "error out"=w538:errorcluster)  [unwired: 2 out]
                  }
                  event "Standby\n2": Value Change {
                    n79 = event-data() -> ()  [unwired: 1 in, 1 out]
                    n80 = flat-sequence {
                      tunnel: [w579] -> w570
                      tunnel: w570 -> [w583]
                      tunnel: w568 -> [w582]
                      tunnel: [w581] -> w566
                      tunnel: [w580] -> w567
                      frame #0 {
                        n81 = local read "Standby\n2"() -> (w573:bool)
                        n82 = Select(t=TRUE, s=w573, f=FALSE) -> (s? t:f=w572:bool)
                        n83 = property on="Standby\n2" class="Bool (strict)"("Blinking"=w572) -> ()  [unwired: 2 in, 2 out]
                      }
                      frame #1 {
                        n84 = local read "Standby\n2"() -> (w577:bool)
                        n85 = Select(t="*D03", s=w577, f="*E03") -> (s? t:f=w579:string)
                      }
                      frame #2 {
                        n86 = Unbundle(w582) -> ("VISA resource name out"=w584:refnum<visa-resource-name>, "error out"=w586:errorcluster, "Delay (ms) 2"=w585:u32, "Write/\nRead \n\n2"=w587:bool)
                        n87 = call "I3252_Comm_Interface.vi"("VISA resource name in"=w584, "error in"=w586, "Delay (ms)"=w585, "Write"=w587, "String to Write"=w583, "Read"=w587) -> ("VISA resource name out"=w580:refnum<visa-resource-name>, "error out"=w581:errorcluster)  [unwired: 2 in, 1 out]
                      }
                    }
                    n88 = Not(x="Standby\n2") -> (.not. x?=w571:bool)
                    n89 = Unbundle(w565) -> ("VISA resource name out"=w564:refnum<visa-resource-name>, "error out"=w563:errorcluster)  [unwired: 2 out]
                  }
                  event "Set Command": Value Change {
                    n90 = event-data() -> ()  [unwired: 1 in, 1 out]
                    n91 = stacked-sequence {
                      tunnel: w593 -> [_ w600 _]
                      tunnel: [_ w599 _] -> w592
                      tunnel: [_ w598 _] -> w591
                      frame #0 {
                        n92 = property on="Set Command" class="Bool"("Blinking"=TRUE) -> ()  [unwired: 2 in, 2 out]
                        n93 = property on="ON" class="Bool (strict)"("Blinking"=FALSE) -> ()  [unwired: 2 in, 2 out]
                      }
                      frame #1 {
                        n94 = flat-sequence {
                          tunnel: [w605] -> w602
                          tunnel: [w608] -> w601
                          tunnel: w602 -> [w609]
                          tunnel: w600 -> [w610]
                          tunnel: [w607] -> w599
                          tunnel: [w606] -> w598
                          tunnel: w601 -> [w615]
                          frame #0 {
                            n95 = Concatenate Strings("*", "Command input") -> (w605:string)
                          }
                          frame #1 {
                            n96 = Unbundle(w610) -> ("VISA resource name out"=w614:refnum<visa-resource-name>, "error out"=w612:errorcluster, "Delay (ms)"=w613:u32, "Write/\nRead"=w611:bool)
                            n97 = call "I3252_Comm_Interface.vi"("VISA resource name in"=w614, "error in"=w612, "Delay (ms)"=w613, "Write"=w611, "String to Write"=w609, "Read"=w611) -> ("VISA resource name out"=w607:refnum<visa-resource-name>, "error out"=w606:errorcluster, "Read String"=w608:string)  [unwired: 2 in]
                          }
                          frame #2 {
                            "Command output" <- w615
                          }
                        }
                      }
                      frame #2 {
                        n98 = property on="Set Command" class="Bool"("Blinking"=FALSE) -> ()  [unwired: 2 in, 2 out]
                      }
                    }
                    n99 = Not(x="Set Command") -> (.not. x?=w595:bool)
                    n100 = Unbundle(w590) -> ("VISA resource name out"=w589:refnum<visa-resource-name>, "error out"=w588:errorcluster)  [unwired: 2 out]
                  }
                  event "Set Command\n\n 2": Value Change {
                    n101 = event-data() -> ()  [unwired: 1 in, 1 out]
                    n102 = stacked-sequence {
                      tunnel: w622 -> [_ w629 _]
                      tunnel: [_ w628 _] -> w620
                      tunnel: [_ w627 _] -> w619
                      frame #0 {
                        n103 = property on="Set Command\n\n 2" class="Bool"("Blinking"=TRUE) -> ()  [unwired: 2 in, 2 out]
                        n104 = property on="ON 2" class="Bool (strict)"("Blinking"=FALSE) -> ()  [unwired: 2 in, 2 out]
                      }
                      frame #1 {
                        n105 = flat-sequence {
                          tunnel: [w634] -> w631
                          tunnel: [w637] -> w630
                          tunnel: w631 -> [w638]
                          tunnel: w629 -> [w639]
                          tunnel: [w636] -> w628
                          tunnel: [w635] -> w627
                          tunnel: w630 -> [w644]
                          frame #0 {
                            n106 = Concatenate Strings("*", "Command input 2") -> (w634:string)
                          }
                          frame #1 {
                            n107 = Unbundle(w639) -> ("VISA resource name out"=w643:refnum<visa-resource-name>, "error out"=w641:errorcluster, "Delay (ms) 2"=w642:u32, "Write/\nRead \n\n2"=w640:bool)
                            n108 = call "I3252_Comm_Interface.vi"("VISA resource name in"=w643, "error in"=w641, "Delay (ms)"=w642, "Write"=w640, "String to Write"=w638, "Read"=w640) -> ("VISA resource name out"=w636:refnum<visa-resource-name>, "error out"=w635:errorcluster, "Read String"=w637:string)  [unwired: 2 in]
                          }
                          frame #2 {
                            "Command output 2" <- w644
                          }
                        }
                      }
                      frame #2 {
                        n109 = property on="Set Command\n\n 2" class="Bool"("Blinking"=FALSE) -> ()  [unwired: 2 in, 2 out]
                      }
                    }
                    n110 = Not(x="Set Command\n\n 2") -> (.not. x?=w624:bool)
                    n111 = Unbundle(w621) -> ("VISA resource name out"=w618:refnum<visa-resource-name>, "error out"=w617:errorcluster)  [unwired: 2 out]
                  }
                  event "Reset\nSTOP": Value Change {
                    n112 = event-data() -> ()  [unwired: 1 in, 1 out]
                    n113 = stacked-sequence {
                      tunnel: [_ w660 _] -> w650
                      tunnel: [_ w659 _] -> w651
                      tunnel: w649 -> [_ w657 _]
                      frame #0 {
                        n114 = property on="Reset\nSTOP" class="Bool"("Blinking"=TRUE) -> ()  [unwired: 2 in, 2 out]
                        n115 = property on="ON" class="Bool (strict)"("Blinking"=FALSE) -> ()  [unwired: 2 in, 2 out]
                      }
                      frame #1 {
                        n116 = for {
                          N: 2 -> [_]
                          tunnel: [w666] -> w660
                          tunnel: [w665] -> w659
                          tunnel: w657 -> [w664]
                          i -> [w662]
                          n117 = flat-sequence {
                            tunnel: w662 -> [w668]
                            tunnel: [w667] -> w663
                            tunnel: [w673] -> w666
                            tunnel: [w674] -> w665
                            tunnel: w664 -> [w675]
                            tunnel: w663 -> [w672]
                            tunnel: [w671] -> w661
                            tunnel: w662 -> [w681]
                            tunnel: w661 -> [w680]
                            frame #0 {
                              n118 = case shown="0, Default" w668 {
                                tunnel: ["*Z02" "*G01"] -> w667
                                frame 0, Default {
                                }
                                frame 1 {
                                }
                              }
                            }
                            frame #1 {
                              n119 = Unbundle(w675) -> ("VISA resource name out"=w676:refnum<visa-resource-name>, "error out"=w678:errorcluster, "Delay (ms)"=w677:u32, "Write/\nRead"=w679:bool)
                              n120 = call "I3252_Comm_Interface.vi"("VISA resource name in"=w676, "error in"=w678, "Delay (ms)"=w677, "Write"=w679, "String to Write"=w672, "Read"=w679) -> ("VISA resource name out"=w674:refnum<visa-resource-name>, "error out"=w673:errorcluster, "Read String"=w671:string)  [unwired: 2 in]
                            }
                            frame #2 {
                              n121 = case shown="0, Default" w681 {
                                tunnel: w680 -> [_ w683]
                                frame 0, Default {
                                }
                                frame 1 {
                                n122 = call "I3252_Edit_Setpoint.vi"("Read String"=w683) -> ("Setpoint is"=w682:dbl)
                                n123 = local write "SP 1 is (°C)"(w682) -> ()
                                }
                              }
                            }
                          }
                        }
                        n124 = Wait (ms)(milliseconds to wait=u32 4000) -> ()  [unwired: 1 out]
                      }
                      frame #2 {
                        n125 = property on="Reset\nSTOP" class="Bool"("Blinking"=FALSE) -> ()  [unwired: 2 in, 2 out]
                      }
                    }
                    n126 = Not(x="Reset\nSTOP") -> (.not. x?=w653:bool)
                    n127 = Unbundle(w646) -> ("VISA resource name out"=w648:refnum<visa-resource-name>, "error out"=w647:errorcluster)  [unwired: 2 out]
                  }
                  event "Reset\nSTOP 2": Value Change {
                    n128 = event-data() -> ()  [unwired: 1 in, 1 out]
                    n129 = stacked-sequence {
                      tunnel: [_ w699 _] -> w688
                      tunnel: [_ w698 _] -> w689
                      tunnel: w690 -> [_ w696 _]
                      frame #0 {
                        n130 = property on="Reset\nSTOP 2" class="Bool"("Blinking"=TRUE) -> ()  [unwired: 2 in, 2 out]
                        n131 = property on="ON 2" class="Bool (strict)"("Blinking"=FALSE) -> ()  [unwired: 2 in, 2 out]
                      }
                      frame #1 {
                        n132 = for {
                          N: 2 -> [_]
                          tunnel: [w705] -> w699
                          tunnel: [w704] -> w698
                          tunnel: w696 -> [w703]
                          i -> [w701]
                          n133 = flat-sequence {
                            tunnel: w701 -> [w707]
                            tunnel: [w706] -> w702
                            tunnel: [w712] -> w705
                            tunnel: [w713] -> w704
                            tunnel: w703 -> [w714]
                            tunnel: w702 -> [w711]
                            tunnel: [w710] -> w700
                            tunnel: w701 -> [w720]
                            tunnel: w700 -> [w719]
                            frame #0 {
                              n134 = case shown="0, Default" w707 {
                                tunnel: ["*Z02" "*G01"] -> w706
                                frame 0, Default {
                                }
                                frame 1 {
                                }
                              }
                            }
                            frame #1 {
                              n135 = Unbundle(w714) -> ("VISA resource name out"=w715:refnum<visa-resource-name>, "error out"=w717:errorcluster, "Delay (ms) 2"=w716:u32, "Write/\nRead \n\n2"=w718:bool)
                              n136 = call "I3252_Comm_Interface.vi"("VISA resource name in"=w715, "error in"=w717, "Delay (ms)"=w716, "Write"=w718, "String to Write"=w711, "Read"=w718) -> ("VISA resource name out"=w713:refnum<visa-resource-name>, "error out"=w712:errorcluster, "Read String"=w710:string)  [unwired: 2 in]
                            }
                            frame #2 {
                              n137 = case shown="1" w720 {
                                tunnel: w719 -> [_ w722]
                                frame 0, Default {
                                }
                                frame 1 {
                                n138 = call "I3252_Edit_Setpoint.vi"("Read String"=w722) -> ("Setpoint is"=w721:dbl)
                                n139 = local write "SP 2 is (°C)"(w721) -> ()
                                }
                              }
                            }
                          }
                        }
                        n140 = Wait (ms)(milliseconds to wait=u32 4000) -> ()  [unwired: 1 out]
                      }
                      frame #2 {
                        n141 = property on="Reset\nSTOP 2" class="Bool"("Blinking"=FALSE) -> ()  [unwired: 2 in, 2 out]
                      }
                    }
                    n142 = Not(x="Reset\nSTOP 2") -> (.not. x?=w692:bool)
                    n143 = Unbundle(w687) -> ("VISA resource name out"=w686:refnum<visa-resource-name>, "error out"=w685:errorcluster)  [unwired: 2 out]
                  }
                  event "Auto Tune": Value Change {
                    n144 = event-data() -> ()  [unwired: 1 in, 1 out]
                    n145 = stacked-sequence {
                      tunnel: w729 -> [_ w736 w781]
                      tunnel: [_ w735 _] -> w728
                      tunnel: [_ w734 _] -> w727
                      frame #0 {
                        n146 = property on="Auto Tune" class="Bool"("Blinking"=TRUE) -> ()  [unwired: 2 in, 2 out]
                        n147 = property on="ON" class="Bool (strict)"("Blinking"=FALSE) -> ()  [unwired: 2 in, 2 out]
                      }
                      frame #1 {
                        n148 = for {
                          N: 4 -> [_]
                          tunnel: [w741] -> w734
                          tunnel: [w740] -> w735
                          tunnel: w736 -> [w739]
                          i -> [w744]
                          n149 = flat-sequence {
                            tunnel: w744 -> [w746]
                            tunnel: [w745] -> w742
                            tunnel: w742 -> [w761]
                            tunnel: [w760] -> w743
                            tunnel: [w763] -> w741
                            tunnel: [w762] -> w740
                            tunnel: w739 -> [w759]
                            tunnel: w744 -> [w769]
                            tunnel: w743 -> [w768]
                            frame #0 {
                              n150 = case shown="0, Default" w746 {
                                tunnel: ["*V01" w749 "*W0C35" "*Z02"] -> w745
                                frame 0, Default {
                                }
                                frame 1 {
                                n151 = local read "(°C)"() -> (w748:dbl)
                                n152 = Add(x=20.0, y=w748) -> (x+y=w755:dbl)
                                n153 = Multiply(x=10.0, y=w755) -> (x*y=w752:dbl)
                                n154 = Number To Hexadecimal String(1:i16 5 ("width (-)"), 2:w752) -> (0:w751:string)
                                n155 = Concatenate Strings("*W012", w751) -> (w749:string)
                                }
                                frame 2 {
                                # "35 hex = \n00110101 bin"
                                }
                                frame 3 {
                                }
                              }
                            }
                            frame #1 {
                              n156 = Unbundle(w759) -> ("VISA resource name out"=w767:refnum<visa-resource-name>, "error out"=w765:errorcluster, "Delay (ms)"=w766:u32, "Write/\nRead"=w764:bool)
                              n157 = call "I3252_Comm_Interface.vi"("VISA resource name in"=w767, "error in"=w765, "Delay (ms)"=w766, "Write"=w764, "String to Write"=w761, "Read"=w764) -> ("VISA resource name out"=w763:refnum<visa-resource-name>, "error out"=w762:errorcluster, "Read String"=w760:string)  [unwired: 2 in]
                            }
                            frame #2 {
                              n158 = case shown="0, Default" w769 {
                                tunnel: w768 -> [w771]
                                frame 0, Default {
                                n159 = call <vilib>:"Space Constant.vi"() -> ("String"=w774:string)
                                n160 = Search/Split String(string=w771, search string/char (-)=w774) -> (match + rest of string=w773:string)  [unwired: 1 in, 2 out]
                                n161 = Fract/Exp String To Number(use system decimal point (T)=FALSE, string=w773) -> (number=w770:dbl)  [unwired: 2 in, 1 out]
                                n162 = local write "(°C)"(w770) -> ()
                                }
                              }
                            }
                          }
                        }
                        n163 = Wait (ms)(milliseconds to wait=u32 45000) -> ()  [unwired: 1 out]
                      }
                      frame #2 {
                        n164 = Unbundle(w781) -> ("VISA resource name out"=w780:refnum<visa-resource-name>, "error out"=w778:errorcluster, "Delay (ms)"=w779:u32, "Write/\nRead"=w777:bool)
                        n165 = property on="Auto Tune" class="Bool"("Blinking"=FALSE) -> ()  [unwired: 2 in, 2 out]
                        n166 = call "I3252_Comm_Interface.vi"("VISA resource name in"=w780, "error in"=w778, "Delay (ms)"=w779, "Write"=w777, "String to Write"="*W01200000", "Read"=w777) -> ()  [unwired: 2 in, 3 out]
                      }
                    }
                    n167 = Not(x="Auto Tune") -> (.not. x?=w730:bool)
                    n168 = Unbundle(w726) -> ("VISA resource name out"=w725:refnum<visa-resource-name>, "error out"=w724:errorcluster)  [unwired: 2 out]
                  }
                  event "Auto Tune 2": Value Change {
                    n169 = event-data() -> ()  [unwired: 1 in, 1 out]
                    n170 = stacked-sequence {
                      tunnel: w782 -> [_ w794 w839]
                      tunnel: [_ w793 _] -> w786
                      tunnel: [_ w792 _] -> w787
                      frame #0 {
                        n171 = property on="Auto Tune 2" class="Bool"("Blinking"=TRUE) -> ()  [unwired: 2 in, 2 out]
                        n172 = property on="ON" class="Bool (strict)"("Blinking"=FALSE) -> ()  [unwired: 2 in, 2 out]
                      }
                      frame #1 {
                        n173 = for {
                          N: 4 -> [_]
                          tunnel: [w799] -> w792
                          tunnel: [w798] -> w793
                          tunnel: w794 -> [w797]
                          i -> [w802]
                          n174 = flat-sequence {
                            tunnel: w802 -> [w804]
                            tunnel: [w803] -> w800
                            tunnel: w800 -> [w819]
                            tunnel: [w818] -> w801
                            tunnel: [w821] -> w799
                            tunnel: [w820] -> w798
                            tunnel: w797 -> [w817]
                            tunnel: w802 -> [w827]
                            tunnel: w801 -> [w826]
                            frame #0 {
                              n175 = case shown="1" w804 {
                                tunnel: ["*V01" w807 "*W0C35" "*Z02"] -> w803
                                frame 0, Default {
                                }
                                frame 1 {
                                n176 = local read "(°C) 2"() -> (w806:dbl)
                                n177 = Add(x=20.0, y=w806) -> (x+y=w813:dbl)
                                n178 = Multiply(x=10.0, y=w813) -> (x*y=w810:dbl)
                                n179 = Number To Hexadecimal String(1:i16 5 ("width (-)"), 2:w810) -> (0:w809:string)
                                n180 = Concatenate Strings("*W012", w809) -> (w807:string)
                                }
                                frame 2 {
                                # "35 hex = \n00110101 bin"
                                }
                                frame 3 {
                                }
                              }
                            }
                            frame #1 {
                              n181 = Unbundle(w817) -> ("VISA resource name out"=w825:refnum<visa-resource-name>, "error out"=w823:errorcluster, "Delay (ms) 2"=w824:u32, "Write/\nRead \n\n2"=w822:bool)
                              n182 = call "I3252_Comm_Interface.vi"("VISA resource name in"=w825, "error in"=w823, "Delay (ms)"=w824, "Write"=w822, "String to Write"=w819, "Read"=w822) -> ("VISA resource name out"=w821:refnum<visa-resource-name>, "error out"=w820:errorcluster, "Read String"=w818:string)  [unwired: 2 in]
                            }
                            frame #2 {
                              n183 = case shown="0, Default" w827 {
                                tunnel: w826 -> [w829]
                                frame 0, Default {
                                n184 = call <vilib>:"Space Constant.vi"() -> ("String"=w832:string)
                                n185 = Search/Split String(string=w829, search string/char (-)=w832) -> (match + rest of string=w831:string)  [unwired: 1 in, 2 out]
                                n186 = Fract/Exp String To Number(use system decimal point (T)=FALSE, string=w831) -> (number=w828:dbl)  [unwired: 2 in, 1 out]
                                n187 = local write "(°C) 2"(w828) -> ()
                                }
                              }
                            }
                          }
                        }
                        n188 = Wait (ms)(milliseconds to wait=u32 45000) -> ()  [unwired: 1 out]
                      }
                      frame #2 {
                        n189 = Unbundle(w839) -> ("VISA resource name out"=w838:refnum<visa-resource-name>, "error out"=w836:errorcluster, "Delay (ms) 2"=w837:u32, "Write/\nRead \n\n2"=w835:bool)
                        n190 = property on="Auto Tune 2" class="Bool"("Blinking"=FALSE) -> ()  [unwired: 2 in, 2 out]
                        n191 = call "I3252_Comm_Interface.vi"("VISA resource name in"=w838, "error in"=w836, "Delay (ms)"=w837, "Write"=w835, "String to Write"="*W01200000", "Read"=w835) -> ()  [unwired: 2 in, 3 out]
                      }
                    }
                    n192 = Not(x="Auto Tune 2") -> (.not. x?=w788:bool)
                    n193 = Unbundle(w783) -> ("VISA resource name out"=w785:refnum<visa-resource-name>, "error out"=w784:errorcluster)  [unwired: 2 out]
                  }
                  event "Write LOW/HI": Value Change {
                    n194 = event-data() -> ()  [unwired: 1 in, 1 out]
                    n195 = stacked-sequence {
                      tunnel: [_ w852 _] -> w845
                      tunnel: [_ w851 _] -> w844
                      tunnel: w843 -> [_ w850 _]
                      frame #0 {
                        n196 = property on="Write LOW/HI" class="Bool"("Blinking"=TRUE) -> ()  [unwired: 2 in, 2 out]
                        n197 = property on="ON" class="Bool (strict)"("Blinking"=FALSE) -> ()  [unwired: 2 in, 2 out]
                      }
                      frame #1 {
                        n198 = for {
                          N: 4 -> [_]
                          tunnel: [w856] -> w852
                          tunnel: [w855] -> w851
                          tunnel: w850 -> [w854]
                          i -> [w858]
                          n199 = flat-sequence {
                            tunnel: w858 -> [w860]
                            tunnel: [w861] -> w857
                            tunnel: w857 -> [w875]
                            tunnel: [w876] -> w859
                            tunnel: [w878] -> w856
                            tunnel: [w877] -> w855
                            tunnel: w854 -> [w874]
                            tunnel: w859 -> [w884]
                            tunnel: w858 -> [w883]
                            frame #0 {
                              n200 = case shown="0, Default" w860 {
                                tunnel: [w863 w869 "*R27" "*R28"] -> w861
                                frame 0, Default {
                                n201 = Number To Hexadecimal String(1:i16 2 ("width (-)"), 2:"% LOW Sollwert") -> (0:w864:string)
                                n202 = Concatenate Strings("*W27", w864) -> (w863:string)
                                }
                                frame 1 {
                                n203 = Number To Hexadecimal String(1:i16 2 ("width (-)"), 2:"% High Sollwert") -> (0:w870:string)
                                n204 = Concatenate Strings("*W28", w870) -> (w869:string)
                                }
                                frame 2 {
                                }
                                frame 3 {
                                }
                              }
                            }
                            frame #1 {
                              n205 = Unbundle(w874) -> ("VISA resource name out"=w882:refnum<visa-resource-name>, "error out"=w880:errorcluster, "Delay (ms)"=w881:u32, "Write/\nRead"=w879:bool)
                              n206 = call "I3252_Comm_Interface.vi"("VISA resource name in"=w882, "error in"=w880, "Delay (ms)"=w881, "Write"=w879, "String to Write"=w875, "Read"=w879) -> ("VISA resource name out"=w878:refnum<visa-resource-name>, "error out"=w877:errorcluster, "Read String"=w876:string)  [unwired: 2 in]
                            }
                            frame #2 {
                              n207 = case shown="0, Default" w883 {
                                tunnel: w884 -> [_ w888 w892]
                                frame 0, Default {
                                }
                                frame 2 {
                                n208 = String Subset(string=w888, offset (0)=3) -> (substring=w886:string)  [unwired: 1 in]
                                n209 = Hexadecimal String To Number(string=w886) -> (number=→"% LOW Istwert":u32)  [unwired: 2 in, 1 out]
                                }
                                frame 3 {
                                n210 = String Subset(string=w892, offset (0)=3) -> (substring=w890:string)  [unwired: 1 in]
                                n211 = Hexadecimal String To Number(string=w890) -> (number=→"% HIGH Istwert":u32)  [unwired: 2 in, 1 out]
                                }
                              }
                            }
                          }
                        }
                      }
                      frame #2 {
                        n212 = property on="Write LOW/HI" class="Bool"("Blinking"=FALSE) -> ()  [unwired: 2 in, 2 out]
                      }
                    }
                    n213 = Not(x="Write LOW/HI") -> (.not. x?=w847:bool)
                    n214 = Unbundle(w842) -> ("VISA resource name out"=w841:refnum<visa-resource-name>, "error out"=w840:errorcluster)  [unwired: 2 out]
                  }
                  event "Write LOW/HI 2": Value Change {
                    n215 = event-data() -> ()  [unwired: 1 in, 1 out]
                    n216 = stacked-sequence {
                      tunnel: [_ w906 _] -> w895
                      tunnel: [_ w905 _] -> w894
                      tunnel: w896 -> [_ w904 _]
                      frame #0 {
                        n217 = property on="Write LOW/HI 2" class="Bool"("Blinking"=TRUE) -> ()  [unwired: 2 in, 2 out]
                        n218 = property on="ON 2" class="Bool (strict)"("Blinking"=FALSE) -> ()  [unwired: 2 in, 2 out]
                      }
                      frame #1 {
                        n219 = for {
                          N: 4 -> [_]
                          tunnel: [w910] -> w906
                          tunnel: [w909] -> w905
                          tunnel: w904 -> [w908]
                          i -> [w912]
                          n220 = flat-sequence {
                            tunnel: w912 -> [w914]
                            tunnel: [w915] -> w911
                            tunnel: w911 -> [w929]
                            tunnel: [w930] -> w913
                            tunnel: [w932] -> w910
                            tunnel: [w931] -> w909
                            tunnel: w908 -> [w928]
                            tunnel: w913 -> [w938]
                            tunnel: w912 -> [w937]
                            frame #0 {
                              n221 = case shown="0, Default" w914 {
                                tunnel: [w918 w923 "*R27" "*R28"] -> w915
                                frame 0, Default {
                                n222 = Number To Hexadecimal String(1:i16 2 ("width (-)"), 2:"% LOW Sollwert 2") -> (0:w919:string)
                                n223 = Concatenate Strings("*W27", w919) -> (w918:string)
                                }
                                frame 1 {
                                n224 = Number To Hexadecimal String(1:i16 2 ("width (-)"), 2:"% High Sollwert 2") -> (0:w924:string)
                                n225 = Concatenate Strings("*W28", w924) -> (w923:string)
                                }
                                frame 2 {
                                }
                                frame 3 {
                                }
                              }
                            }
                            frame #1 {
                              n226 = Unbundle(w928) -> ("VISA resource name out"=w936:refnum<visa-resource-name>, "error out"=w934:errorcluster, "Delay (ms) 2"=w935:u32, "Write/\nRead \n\n2"=w933:bool)
                              n227 = call "I3252_Comm_Interface.vi"("VISA resource name in"=w936, "error in"=w934, "Delay (ms)"=w935, "Write"=w933, "String to Write"=w929, "Read"=w933) -> ("VISA resource name out"=w932:refnum<visa-resource-name>, "error out"=w931:errorcluster, "Read String"=w930:string)  [unwired: 2 in]
                            }
                            frame #2 {
                              n228 = case shown="3" w937 {
                                tunnel: w938 -> [_ w942 w946]
                                frame 0, Default {
                                }
                                frame 2 {
                                n229 = String Subset(string=w942, offset (0)=3) -> (substring=w940:string)  [unwired: 1 in]
                                n230 = Hexadecimal String To Number(string=w940) -> (number=→"% LOW Istwert 2":u32)  [unwired: 2 in, 1 out]
                                }
                                frame 3 {
                                n231 = String Subset(string=w946, offset (0)=3) -> (substring=w944:string)  [unwired: 1 in]
                                n232 = Hexadecimal String To Number(string=w944) -> (number=→"% HIGH Istwert 2":u32)  [unwired: 2 in, 1 out]
                                }
                              }
                            }
                          }
                        }
                      }
                      frame #2 {
                        n233 = property on="Write LOW/HI 2" class="Bool"("Blinking"=FALSE) -> ()  [unwired: 2 in, 2 out]
                      }
                    }
                    n234 = Not(x="Write LOW/HI 2") -> (.not. x?=w901:bool)
                    n235 = Unbundle(w899) -> ("VISA resource name out"=w898:refnum<visa-resource-name>, "error out"=w897:errorcluster)  [unwired: 2 out]
                  }
                  event "Set PID": Value Change {
                    n236 = event-data() -> ()  [unwired: 1 in, 1 out]
                    n237 = stacked-sequence {
                      tunnel: w953 -> [_ w960 _]
                      tunnel: [_ w959 _] -> w952
                      tunnel: [_ w958 _] -> w951
                      frame #0 {
                        n238 = property on="Set PID" class="Bool"("Blinking"=TRUE) -> ()  [unwired: 2 in, 2 out]
                        n239 = property on="ON" class="Bool (strict)"("Blinking"=FALSE) -> ()  [unwired: 2 in, 2 out]
                      }
                      frame #1 {
                        n240 = for {
                          N: 6 -> [_]
                          tunnel: w960 -> [w964]
                          tunnel: [w963] -> w959
                          tunnel: [w962] -> w958
                          i -> [w966]
                          n241 = flat-sequence {
                            tunnel: w966 -> [w968]
                            tunnel: [w969] -> w965
                            tunnel: w965 -> [w1010]
                            tunnel: [w1006] -> w967
                            tunnel: w964 -> [w1009]
                            tunnel: [w1008] -> w962
                            tunnel: [w1007] -> w963
                            tunnel: w967 -> [w1016]
                            tunnel: w966 -> [w1015]
                            frame #0 {
                              n242 = case shown="2" w968 {
                                tunnel: [w976 w984 w992 w994 w998 w1002] -> w969
                                frame 0, Default {
                                n243 = local read "RAM"() -> (w970:bool)
                                n244 = Number To Hexadecimal String(1:i16 4 ("width (-)"), 2:"P (PB1) Sollwert") -> (0:w977:string)
                                n245 = Select(t="*P17", s=w970, f="*W17") -> (s? t:f=w971:string)
                                n246 = Concatenate Strings(w971, w977) -> (w976:string)
                                }
                                frame 1 {
                                n247 = local read "RAM"() -> (w978:bool)
                                n248 = Number To Hexadecimal String(1:i16 4 ("width (-)"), 2:"I ( Reset1) Sollwert") -> (0:w985:string)
                                n249 = Select(t="*P18", s=w978, f="*W18") -> (s? t:f=w980:string)
                                n250 = Concatenate Strings(w980, w985) -> (w984:string)
                                }
                                frame 2 {
                                n251 = local read "RAM"() -> (w987:bool)
                                n252 = Number To Hexadecimal String(1:i16 4 ("width (-)"), 2:"D (Rate) Sollwert") -> (0:w993:string)
                                n253 = Select(t="*P19", s=w987, f="*W19") -> (s? t:f=w988:string)
                                n254 = Concatenate Strings(w988, w993) -> (w992:string)
                                }
                                frame 3 {
                                n255 = local read "RAM"() -> (w997:bool)
                                n256 = Select(t="*G17", s=w997, f="*R17") -> (s? t:f=w994:string)
                                }
                                frame 4 {
                                n257 = local read "RAM"() -> (w1001:bool)
                                n258 = Select(t="*G18", s=w1001, f="*R18") -> (s? t:f=w998:string)
                                }
                                frame 5 {
                                n259 = local read "RAM"() -> (w1005:bool)
                                n260 = Select(t="*G19", s=w1005, f="*R19") -> (s? t:f=w1002:string)
                                }
                              }
                            }
                            frame #1 {
                              n261 = Unbundle(w1009) -> ("VISA resource name out"=w1014:refnum<visa-resource-name>, "error out"=w1012:errorcluster, "Delay (ms)"=w1013:u32, "Write/\nRead"=w1011:bool)
                              n262 = call "I3252_Comm_Interface.vi"("VISA resource name in"=w1014, "error in"=w1012, "Delay (ms)"=w1013, "Write"=w1011, "String to Write"=w1010, "Read"=w1011) -> ("VISA resource name out"=w1007:refnum<visa-resource-name>, "error out"=w1008:errorcluster, "Read String"=w1006:string)  [unwired: 2 in]
                            }
                            frame #2 {
                              n263 = case shown="4" w1015 {
                                tunnel: w1016 -> [_ w1020 w1024 w1028]
                                frame 0, Default {
                                }
                                frame 3 {
                                n264 = String Subset(string=w1020, offset (0)=3) -> (substring=w1018:string)  [unwired: 1 in]
                                n265 = Hexadecimal String To Number(string=w1018) -> (number=→"P (PB1) Istwert":u32)  [unwired: 2 in, 1 out]
                                }
                                frame 4 {
                                n266 = String Subset(string=w1024, offset (0)=3) -> (substring=w1022:string)  [unwired: 1 in]
                                n267 = Hexadecimal String To Number(string=w1022) -> (number=→"I ( Reset1) Istwert":u32)  [unwired: 2 in, 1 out]
                                }
                                frame 5 {
                                n268 = String Subset(string=w1028, offset (0)=3) -> (substring=w1026:string)  [unwired: 1 in]
                                n269 = Hexadecimal String To Number(string=w1026) -> (number=→"D (Rate) IstWert":u32)  [unwired: 2 in, 1 out]
                                }
                              }
                            }
                          }
                        }
                      }
                      frame #2 {
                        n270 = property on="Set PID" class="Bool"("Blinking"=FALSE) -> ()  [unwired: 2 in, 2 out]
                      }
                    }
                    n271 = Not(x="Set PID") -> (.not. x?=w955:bool)
                    n272 = Unbundle(w950) -> ("VISA resource name out"=w949:refnum<visa-resource-name>, "error out"=w948:errorcluster)  [unwired: 2 out]
                  }
                  event "Set PID 2": Value Change {
                    n273 = event-data() -> ()  [unwired: 1 in, 1 out]
                    n274 = stacked-sequence {
                      tunnel: w1030 -> [_ w1042 _]
                      tunnel: [_ w1041 _] -> w1032
                      tunnel: [_ w1040 _] -> w1031
                      frame #0 {
                        n275 = property on="Set PID 2" class="Bool"("Blinking"=TRUE) -> ()  [unwired: 2 in, 2 out]
                        n276 = property on="ON 2" class="Bool (strict)"("Blinking"=FALSE) -> ()  [unwired: 2 in, 2 out]
                      }
                      frame #1 {
                        n277 = for {
                          N: 6 -> [_]
                          tunnel: w1042 -> [w1046]
                          tunnel: [w1045] -> w1041
                          tunnel: [w1044] -> w1040
                          i -> [w1048]
                          n278 = flat-sequence {
                            tunnel: w1048 -> [w1050]
                            tunnel: [w1051] -> w1047
                            tunnel: w1047 -> [w1092]
                            tunnel: [w1088] -> w1049
                            tunnel: w1046 -> [w1091]
                            tunnel: [w1090] -> w1044
                            tunnel: [w1089] -> w1045
                            tunnel: w1049 -> [w1098]
                            tunnel: w1048 -> [w1097]
                            frame #0 {
                              n279 = case shown="0, Default" w1050 {
                                tunnel: [w1058 w1066 w1074 w1076 w1080 w1084] -> w1051
                                frame 0, Default {
                                n280 = local read "RAM 2"() -> (w1053:bool)
                                n281 = Number To Hexadecimal String(1:i16 4 ("width (-)"), 2:"P (PB1) Sollwert 2") -> (0:w1059:string)
                                n282 = Select(t="*P17", s=w1053, f="*W17") -> (s? t:f=w1054:string)
                                n283 = Concatenate Strings(w1054, w1059) -> (w1058:string)
                                }
                                frame 1 {
                                n284 = local read "RAM 2"() -> (w1061:bool)
                                n285 = Number To Hexadecimal String(1:i16 4 ("width (-)"), 2:"I ( Reset1) Sollwert 2") -> (0:w1067:string)
                                n286 = Select(t="*P18", s=w1061, f="*W18") -> (s? t:f=w1062:string)
                                n287 = Concatenate Strings(w1062, w1067) -> (w1066:string)
                                }
                                frame 2 {
                                n288 = local read "RAM 2"() -> (w1069:bool)
                                n289 = Number To Hexadecimal String(1:i16 4 ("width (-)"), 2:"D (Rate) Sollwert 2") -> (0:w1075:string)
                                n290 = Select(t="*P19", s=w1069, f="*W19") -> (s? t:f=w1070:string)
                                n291 = Concatenate Strings(w1070, w1075) -> (w1074:string)
                                }
                                frame 3 {
                                n292 = local read "RAM"() -> (w1079:bool)
                                n293 = Select(t="*G17", s=w1079, f="*R17") -> (s? t:f=w1076:string)
                                }
                                frame 4 {
                                n294 = local read "RAM"() -> (w1083:bool)
                                n295 = Select(t="*G18", s=w1083, f="*R18") -> (s? t:f=w1080:string)
                                }
                                frame 5 {
                                n296 = local read "RAM"() -> (w1087:bool)
                                n297 = Select(t="*G19", s=w1087, f="*R19") -> (s? t:f=w1084:string)
                                }
                              }
                            }
                            frame #1 {
                              n298 = Unbundle(w1091) -> ("VISA resource name out"=w1096:refnum<visa-resource-name>, "error out"=w1094:errorcluster, "Delay (ms) 2"=w1095:u32, "Write/\nRead \n\n2"=w1093:bool)
                              n299 = call "I3252_Comm_Interface.vi"("VISA resource name in"=w1096, "error in"=w1094, "Delay (ms)"=w1095, "Write"=w1093, "String to Write"=w1092, "Read"=w1093) -> ("VISA resource name out"=w1089:refnum<visa-resource-name>, "error out"=w1090:errorcluster, "Read String"=w1088:string)  [unwired: 2 in]
                            }
                            frame #2 {
                              n300 = case shown="0, Default" w1097 {
                                tunnel: w1098 -> [_ w1102 w1106 w1110]
                                frame 0, Default {
                                }
                                frame 3 {
                                n301 = String Subset(string=w1102, offset (0)=3) -> (substring=w1100:string)  [unwired: 1 in]
                                n302 = Hexadecimal String To Number(string=w1100) -> (number=→"P (PB1) Istwert 2":u32)  [unwired: 2 in, 1 out]
                                }
                                frame 4 {
                                n303 = String Subset(string=w1106, offset (0)=3) -> (substring=w1104:string)  [unwired: 1 in]
                                n304 = Hexadecimal String To Number(string=w1104) -> (number=→"I ( Reset1) Istwert 2":u32)  [unwired: 2 in, 1 out]
                                }
                                frame 5 {
                                n305 = String Subset(string=w1110, offset (0)=3) -> (substring=w1108:string)  [unwired: 1 in]
                                n306 = Hexadecimal String To Number(string=w1108) -> (number=→"D (Rate) IstWert 2":u32)  [unwired: 2 in, 1 out]
                                }
                              }
                            }
                          }
                        }
                      }
                      frame #2 {
                        n307 = property on="Set PID 2" class="Bool"("Blinking"=FALSE) -> ()  [unwired: 2 in, 2 out]
                      }
                    }
                    n308 = Not(x="Set PID 2") -> (.not. x?=w1037:bool)
                    n309 = Unbundle(w1035) -> ("VISA resource name out"=w1034:refnum<visa-resource-name>, "error out"=w1033:errorcluster)  [unwired: 2 out]
                  }
                  event "Get Values": Value Change {
                    n310 = event-data() -> ()  [unwired: 1 in, 1 out]
                    n311 = stacked-sequence {
                      tunnel: w1117 -> [_ w1124 _]
                      tunnel: [_ w1123 _] -> w1116
                      tunnel: [_ w1122 _] -> w1115
                      frame #0 {
                        n312 = property on="Get Values" class="Bool"("Blinking"=TRUE) -> ()  [unwired: 2 in, 2 out]
                        n313 = property on="ON" class="Bool (strict)"("Blinking"=FALSE) -> ()  [unwired: 2 in, 2 out]
                      }
                      frame #1 {
                        n314 = for {
                          N: 6 -> [_]
                          tunnel: w1124 -> [w1128]
                          tunnel: [w1127] -> w1123
                          tunnel: [w1126] -> w1122
                          i -> [w1130]
                          n315 = flat-sequence {
                            tunnel: w1130 -> [w1132]
                            tunnel: [w1133] -> w1129
                            tunnel: w1129 -> [w1155]
                            tunnel: [w1156] -> w1131
                            tunnel: w1128 -> [w1154]
                            tunnel: [w1153] -> w1126
                            tunnel: [w1152] -> w1127
                            tunnel: w1131 -> [w1162]
                            tunnel: w1130 -> [w1161]
                            frame #0 {
                              n316 = case shown="0, Default" w1132 {
                                tunnel: [w1136 w1140 w1144 "*R27" "*R28" w1150] -> w1133
                                frame 0, Default {
                                n317 = local read "RAM"() -> (w1137:bool)
                                n318 = Select(t="*G17", s=w1137, f="*R17") -> (s? t:f=w1136:string)
                                }
                                frame 1 {
                                n319 = local read "RAM"() -> (w1141:bool)
                                n320 = Select(t="*G18", s=w1141, f="*R18") -> (s? t:f=w1140:string)
                                }
                                frame 2 {
                                n321 = local read "RAM"() -> (w1145:bool)
                                n322 = Select(t="*G19", s=w1145, f="*R19") -> (s? t:f=w1144:string)
                                }
                                frame 3 {
                                }
                                frame 4 {
                                }
                                frame 5 {
                                n323 = local read "RAM"() -> (w1151:bool)
                                n324 = Select(t="*G01", s=w1151, f="*R01") -> (s? t:f=w1150:string)
                                }
                              }
                            }
                            frame #1 {
                              n325 = Unbundle(w1154) -> ("VISA resource name out"=w1160:refnum<visa-resource-name>, "error out"=w1158:errorcluster, "Delay (ms)"=w1159:u32, "Write/\nRead"=w1157:bool)
                              n326 = call "I3252_Comm_Interface.vi"("VISA resource name in"=w1160, "error in"=w1158, "Delay (ms)"=w1159, "Write"=w1157, "String to Write"=w1155, "Read"=w1157) -> ("VISA resource name out"=w1152:refnum<visa-resource-name>, "error out"=w1153:errorcluster, "Read String"=w1156:string)  [unwired: 2 in]
                            }
                            frame #2 {
                              n327 = case shown="1" w1161 {
                                tunnel: w1162 -> [w1164 w1168 w1172 w1176 w1180 w1184]
                                frame 0, Default {
                                n328 = String Subset(string=w1164, offset (0)=3) -> (substring=w1165:string)  [unwired: 1 in]
                                n329 = Hexadecimal String To Number(string=w1165) -> (number=w1163:u32)  [unwired: 2 in, 1 out]
                                n330 = local write "P (PB1) Sollwert"(w1163) -> ()
                                n331 = local write "P (PB1) Istwert"(w1163) -> ()
                                }
                                frame 1 {
                                n332 = String Subset(string=w1168, offset (0)=3) -> (substring=w1169:string)  [unwired: 1 in]
                                n333 = Hexadecimal String To Number(string=w1169) -> (number=w1167:u32)  [unwired: 2 in, 1 out]
                                n334 = local write "I ( Reset1) Sollwert"(w1167) -> ()
                                n335 = local write "I ( Reset1) Istwert"(w1167) -> ()
                                }
                                frame 2 {
                                n336 = String Subset(string=w1172, offset (0)=3) -> (substring=w1173:string)  [unwired: 1 in]
                                n337 = Hexadecimal String To Number(string=w1173) -> (number=w1171:u32)  [unwired: 2 in, 1 out]
                                n338 = local write "D (Rate) Sollwert"(w1171) -> ()
                                n339 = local write "D (Rate) IstWert"(w1171) -> ()
                                }
                                frame 3 {
                                n340 = String Subset(string=w1176, offset (0)=3) -> (substring=w1177:string)  [unwired: 1 in]
                                n341 = Hexadecimal String To Number(string=w1177) -> (number=w1175:u32)  [unwired: 2 in, 1 out]
                                n342 = local write "% LOW Istwert"(w1175) -> ()
                                n343 = local write "% LOW Sollwert"(w1175) -> ()
                                }
                                frame 4 {
                                n344 = String Subset(string=w1180, offset (0)=3) -> (substring=w1181:string)  [unwired: 1 in]
                                n345 = Hexadecimal String To Number(string=w1181) -> (number=w1179:u32)  [unwired: 2 in, 1 out]
                                n346 = local write "% High Sollwert"(w1179) -> ()
                                n347 = local write "% HIGH Istwert"(w1179) -> ()
                                }
                                frame 5 {
                                n348 = call "I3252_Edit_Setpoint.vi"("Read String"=w1184) -> ("Setpoint is"=w1183:dbl)
                                n349 = local write "SP 1 is (°C)"(w1183) -> ()
                                }
                              }
                            }
                          }
                        }
                      }
                      frame #2 {
                        n350 = property on="Get Values" class="Bool"("Blinking"=FALSE) -> ()  [unwired: 2 in, 2 out]
                      }
                    }
                    n351 = Not(x="Get Values") -> (.not. x?=w1119:bool)
                    n352 = Unbundle(w1114) -> ("VISA resource name out"=w1113:refnum<visa-resource-name>, "error out"=w1112:errorcluster)  [unwired: 2 out]
                  }
                  event "Get Values 2": Value Change {
                    n353 = event-data() -> ()  [unwired: 1 in, 1 out]
                    n354 = stacked-sequence {
                      tunnel: w1188 -> [_ w1198 _]
                      tunnel: [_ w1197 _] -> w1187
                      tunnel: [_ w1196 _] -> w1186
                      frame #0 {
                        n355 = property on="Get Values 2" class="Bool"("Blinking"=TRUE) -> ()  [unwired: 2 in, 2 out]
                        n356 = property on="ON 2" class="Bool (strict)"("Blinking"=FALSE) -> ()  [unwired: 2 in, 2 out]
                      }
                      frame #1 {
                        n357 = for {
                          N: 6 -> [_]
                          tunnel: w1198 -> [w1202]
                          tunnel: [w1201] -> w1197
                          tunnel: [w1200] -> w1196
                          i -> [w1204]
                          n358 = flat-sequence {
                            tunnel: w1204 -> [w1206]
                            tunnel: [w1207] -> w1203
                            tunnel: w1203 -> [w1229]
                            tunnel: [w1230] -> w1205
                            tunnel: w1202 -> [w1228]
                            tunnel: [w1227] -> w1200
                            tunnel: [w1226] -> w1201
                            tunnel: w1205 -> [w1236]
                            tunnel: w1204 -> [w1235]
                            frame #0 {
                              n359 = case shown="1" w1206 {
                                tunnel: [w1210 w1214 w1218 "*R27" "*R28" w1224] -> w1207
                                frame 0, Default {
                                n360 = local read "RAM 2"() -> (w1211:bool)
                                n361 = Select(t="*G17", s=w1211, f="*R17") -> (s? t:f=w1210:string)
                                }
                                frame 1 {
                                n362 = local read "RAM 2"() -> (w1215:bool)
                                n363 = Select(t="*G18", s=w1215, f="*R18") -> (s? t:f=w1214:string)
                                }
                                frame 2 {
                                n364 = local read "RAM 2"() -> (w1219:bool)
                                n365 = Select(t="*G19", s=w1219, f="*R19") -> (s? t:f=w1218:string)
                                }
                                frame 3 {
                                }
                                frame 4 {
                                }
                                frame 5 {
                                n366 = local read "RAM 2"() -> (w1225:bool)
                                n367 = Select(t="*G01", s=w1225, f="*R01") -> (s? t:f=w1224:string)
                                }
                              }
                            }
                            frame #1 {
                              n368 = Unbundle(w1228) -> ("VISA resource name out"=w1234:refnum<visa-resource-name>, "error out"=w1232:errorcluster, "Delay (ms) 2"=w1233:u32, "Write/\nRead \n\n2"=w1231:bool)
                              n369 = call "I3252_Comm_Interface.vi"("VISA resource name in"=w1234, "error in"=w1232, "Delay (ms)"=w1233, "Write"=w1231, "String to Write"=w1229, "Read"=w1231) -> ("VISA resource name out"=w1226:refnum<visa-resource-name>, "error out"=w1227:errorcluster, "Read String"=w1230:string)  [unwired: 2 in]
                            }
                            frame #2 {
                              n370 = case shown="0, Default" w1235 {
                                tunnel: w1236 -> [w1238 w1242 w1246 w1250 w1254 w1258]
                                frame 0, Default {
                                n371 = String Subset(string=w1238, offset (0)=3) -> (substring=w1239:string)  [unwired: 1 in]
                                n372 = Hexadecimal String To Number(string=w1239) -> (number=w1237:u32)  [unwired: 2 in, 1 out]
                                n373 = local write "P (PB1) Sollwert 2"(w1237) -> ()
                                n374 = local write "P (PB1) Istwert 2"(w1237) -> ()
                                }
                                frame 1 {
                                n375 = String Subset(string=w1242, offset (0)=3) -> (substring=w1243:string)  [unwired: 1 in]
                                n376 = Hexadecimal String To Number(string=w1243) -> (number=w1241:u32)  [unwired: 2 in, 1 out]
                                n377 = local write "I ( Reset1) Sollwert 2"(w1241) -> ()
                                n378 = local write "I ( Reset1) Istwert 2"(w1241) -> ()
                                }
                                frame 2 {
                                n379 = String Subset(string=w1246, offset (0)=3) -> (substring=w1247:string)  [unwired: 1 in]
                                n380 = Hexadecimal String To Number(string=w1247) -> (number=w1245:u32)  [unwired: 2 in, 1 out]
                                n381 = local write "D (Rate) Sollwert 2"(w1245) -> ()
                                n382 = local write "D (Rate) IstWert 2"(w1245) -> ()
                                }
                                frame 3 {
                                n383 = String Subset(string=w1250, offset (0)=3) -> (substring=w1251:string)  [unwired: 1 in]
                                n384 = Hexadecimal String To Number(string=w1251) -> (number=w1249:u32)  [unwired: 2 in, 1 out]
                                n385 = local write "% LOW Istwert 2"(w1249) -> ()
                                n386 = local write "% LOW Sollwert 2"(w1249) -> ()
                                }
                                frame 4 {
                                n387 = String Subset(string=w1254, offset (0)=3) -> (substring=w1255:string)  [unwired: 1 in]
                                n388 = Hexadecimal String To Number(string=w1255) -> (number=w1253:u32)  [unwired: 2 in, 1 out]
                                n389 = local write "% High Sollwert 2"(w1253) -> ()
                                n390 = local write "% HIGH Istwert 2"(w1253) -> ()
                                }
                                frame 5 {
                                n391 = call "I3252_Edit_Setpoint.vi"("Read String"=w1258) -> ("Setpoint is"=w1257:dbl)
                                n392 = local write "SP 2 is (°C)"(w1257) -> ()
                                }
                              }
                            }
                          }
                        }
                      }
                      frame #2 {
                        n393 = property on="Get Values 2" class="Bool"("Blinking"=FALSE) -> ()  [unwired: 2 in, 2 out]
                      }
                    }
                    n394 = Not(x="Get Values 2") -> (.not. x?=w1193:bool)
                    n395 = Unbundle(w1189) -> ("VISA resource name out"=w1191:refnum<visa-resource-name>, "error out"=w1190:errorcluster)  [unwired: 2 out]
                  }
                  event "RAM": Value Change {
                    n396 = event-data() -> ()  [unwired: 1 in, 1 out]
                    n397 = stacked-sequence {
                      tunnel: w1265 -> [_ w1272 _]
                      tunnel: [_ w1271 _] -> w1264
                      tunnel: [_ w1270 _] -> w1263
                      frame #0 {
                        n398 = property on="RAM" class="Bool (strict)"("Blinking"=TRUE) -> ()  [unwired: 2 in, 2 out]
                        n399 = property on="ON" class="Bool (strict)"("Blinking"=FALSE) -> ()  [unwired: 2 in, 2 out]
                      }
                      frame #1 {
                        n400 = for {
                          N: 6 -> [_]
                          tunnel: w1272 -> [w1276]
                          tunnel: [w1275] -> w1271
                          tunnel: [w1274] -> w1270
                          i -> [w1278]
                          n401 = flat-sequence {
                            tunnel: w1278 -> [w1280]
                            tunnel: [w1281] -> w1277
                            tunnel: w1277 -> [w1300]
                            tunnel: [w1301] -> w1279
                            tunnel: w1276 -> [w1304]
                            tunnel: [w1303] -> w1274
                            tunnel: [w1302] -> w1275
                            tunnel: w1279 -> [w1310]
                            tunnel: w1278 -> [w1309]
                            frame #0 {
                              n402 = case shown="3" w1280 {
                                tunnel: [w1284 w1288 w1292 "*R27" "*R28" w1298] -> w1281
                                frame 0, Default {
                                n403 = local read "RAM"() -> (w1285:bool)
                                n404 = Select(t="*G17", s=w1285, f="*R17") -> (s? t:f=w1284:string)
                                }
                                frame 1 {
                                n405 = local read "RAM"() -> (w1289:bool)
                                n406 = Select(t="*G18", s=w1289, f="*R18") -> (s? t:f=w1288:string)
                                }
                                frame 2 {
                                n407 = local read "RAM"() -> (w1293:bool)
                                n408 = Select(t="*G19", s=w1293, f="*R19") -> (s? t:f=w1292:string)
                                }
                                frame 3 {
                                }
                                frame 4 {
                                }
                                frame 5 {
                                n409 = local read "RAM"() -> (w1299:bool)
                                n410 = Select(t="*G01", s=w1299, f="*R01") -> (s? t:f=w1298:string)
                                }
                              }
                            }
                            frame #1 {
                              n411 = Unbundle(w1304) -> ("VISA resource name out"=w1308:refnum<visa-resource-name>, "error out"=w1306:errorcluster, "Delay (ms)"=w1307:u32, "Write/\nRead"=w1305:bool)
                              n412 = call "I3252_Comm_Interface.vi"("VISA resource name in"=w1308, "error in"=w1306, "Delay (ms)"=w1307, "Write"=w1305, "String to Write"=w1300, "Read"=w1305) -> ("VISA resource name out"=w1302:refnum<visa-resource-name>, "error out"=w1303:errorcluster, "Read String"=w1301:string)  [unwired: 2 in]
                            }
                            frame #2 {
                              n413 = case shown="5" w1309 {
                                tunnel: w1310 -> [w1312 w1316 w1320 w1324 w1328 w1332]
                                frame 0, Default {
                                n414 = String Subset(string=w1312, offset (0)=3) -> (substring=w1313:string)  [unwired: 1 in]
                                n415 = Hexadecimal String To Number(string=w1313) -> (number=w1311:u32)  [unwired: 2 in, 1 out]
                                n416 = local write "P (PB1) Sollwert"(w1311) -> ()
                                n417 = local write "P (PB1) Istwert"(w1311) -> ()
                                }
                                frame 1 {
                                n418 = String Subset(string=w1316, offset (0)=3) -> (substring=w1317:string)  [unwired: 1 in]
                                n419 = Hexadecimal String To Number(string=w1317) -> (number=w1315:u32)  [unwired: 2 in, 1 out]
                                n420 = local write "I ( Reset1) Sollwert"(w1315) -> ()
                                n421 = local write "I ( Reset1) Istwert"(w1315) -> ()
                                }
                                frame 2 {
                                n422 = String Subset(string=w1320, offset (0)=3) -> (substring=w1321:string)  [unwired: 1 in]
                                n423 = Hexadecimal String To Number(string=w1321) -> (number=w1319:u32)  [unwired: 2 in, 1 out]
                                n424 = local write "D (Rate) IstWert"(w1319) -> ()
                                n425 = local write "D (Rate) Sollwert"(w1319) -> ()
                                }
                                frame 3 {
                                n426 = String Subset(string=w1324, offset (0)=3) -> (substring=w1325:string)  [unwired: 1 in]
                                n427 = Hexadecimal String To Number(string=w1325) -> (number=w1323:u32)  [unwired: 2 in, 1 out]
                                n428 = local write "% LOW Istwert"(w1323) -> ()
                                n429 = local write "% LOW Sollwert"(w1323) -> ()
                                }
                                frame 4 {
                                n430 = String Subset(string=w1328, offset (0)=3) -> (substring=w1329:string)  [unwired: 1 in]
                                n431 = Hexadecimal String To Number(string=w1329) -> (number=w1327:u32)  [unwired: 2 in, 1 out]
                                n432 = local write "% HIGH Istwert"(w1327) -> ()
                                n433 = local write "% High Sollwert"(w1327) -> ()
                                }
                                frame 5 {
                                n434 = call "I3252_Edit_Setpoint.vi"("Read String"=w1332) -> ("Setpoint is"=w1331:dbl)
                                n435 = local write "SP 1 is (°C)"(w1331) -> ()
                                }
                              }
                            }
                          }
                        }
                      }
                      frame #2 {
                        n436 = property on="RAM" class="Bool (strict)"("Blinking"=FALSE) -> ()  [unwired: 2 in, 2 out]
                      }
                    }
                    n437 = Not(x="RAM") -> (.not. x?=w1267:bool)
                    n438 = Unbundle(w1262) -> ("VISA resource name out"=w1261:refnum<visa-resource-name>, "error out"=w1260:errorcluster)  [unwired: 2 out]
                  }
                  event "RAM 2": Value Change {
                    n439 = event-data() -> ()  [unwired: 1 in, 1 out]
                    n440 = stacked-sequence {
                      tunnel: w1336 -> [_ w1346 _]
                      tunnel: [_ w1345 _] -> w1335
                      tunnel: [_ w1344 _] -> w1334
                      frame #0 {
                        n441 = property on="RAM 2" class="Bool (strict)"("Blinking"=TRUE) -> ()  [unwired: 2 in, 2 out]
                        n442 = property on="ON 2" class="Bool (strict)"("Blinking"=FALSE) -> ()  [unwired: 2 in, 2 out]
                      }
                      frame #1 {
                        n443 = for {
                          N: 6 -> [_]
                          tunnel: w1346 -> [w1350]
                          tunnel: [w1349] -> w1345
                          tunnel: [w1348] -> w1344
                          i -> [w1352]
                          n444 = flat-sequence {
                            tunnel: w1352 -> [w1354]
                            tunnel: [w1355] -> w1351
                            tunnel: w1351 -> [w1374]
                            tunnel: [w1375] -> w1353
                            tunnel: w1350 -> [w1378]
                            tunnel: [w1377] -> w1348
                            tunnel: [w1376] -> w1349
                            tunnel: w1353 -> [w1384]
                            tunnel: w1352 -> [w1383]
                            frame #0 {
                              n445 = case shown="5" w1354 {
                                tunnel: [w1358 w1362 w1366 "*R27" "*R28" w1372] -> w1355
                                frame 0, Default {
                                n446 = local read "RAM 2"() -> (w1359:bool)
                                n447 = Select(t="*G17", s=w1359, f="*R17") -> (s? t:f=w1358:string)
                                }
                                frame 1 {
                                n448 = local read "RAM 2"() -> (w1363:bool)
                                n449 = Select(t="*G18", s=w1363, f="*R18") -> (s? t:f=w1362:string)
                                }
                                frame 2 {
                                n450 = local read "RAM 2"() -> (w1367:bool)
                                n451 = Select(t="*G19", s=w1367, f="*R19") -> (s? t:f=w1366:string)
                                }
                                frame 3 {
                                }
                                frame 4 {
                                }
                                frame 5 {
                                n452 = local read "RAM 2"() -> (w1373:bool)
                                n453 = Select(t="*G01", s=w1373, f="*R01") -> (s? t:f=w1372:string)
                                }
                              }
                            }
                            frame #1 {
                              n454 = Unbundle(w1378) -> ("VISA resource name out"=w1382:refnum<visa-resource-name>, "error out"=w1380:errorcluster, "Delay (ms) 2"=w1381:u32, "Write/\nRead \n\n2"=w1379:bool)
                              n455 = call "I3252_Comm_Interface.vi"("VISA resource name in"=w1382, "error in"=w1380, "Delay (ms)"=w1381, "Write"=w1379, "String to Write"=w1374, "Read"=w1379) -> ("VISA resource name out"=w1376:refnum<visa-resource-name>, "error out"=w1377:errorcluster, "Read String"=w1375:string)  [unwired: 2 in]
                            }
                            frame #2 {
                              n456 = case shown="0, Default" w1383 {
                                tunnel: w1384 -> [w1386 w1390 w1394 w1398 w1402 w1406]
                                frame 0, Default {
                                n457 = String Subset(string=w1386, offset (0)=3) -> (substring=w1387:string)  [unwired: 1 in]
                                n458 = Hexadecimal String To Number(string=w1387) -> (number=w1385:u32)  [unwired: 2 in, 1 out]
                                n459 = local write "P (PB1) Sollwert 2"(w1385) -> ()
                                n460 = local write "P (PB1) Istwert 2"(w1385) -> ()
                                }
                                frame 1 {
                                n461 = String Subset(string=w1390, offset (0)=3) -> (substring=w1391:string)  [unwired: 1 in]
                                n462 = Hexadecimal String To Number(string=w1391) -> (number=w1389:u32)  [unwired: 2 in, 1 out]
                                n463 = local write "I ( Reset1) Sollwert 2"(w1389) -> ()
                                n464 = local write "I ( Reset1) Istwert 2"(w1389) -> ()
                                }
                                frame 2 {
                                n465 = String Subset(string=w1394, offset (0)=3) -> (substring=w1395:string)  [unwired: 1 in]
                                n466 = Hexadecimal String To Number(string=w1395) -> (number=w1393:u32)  [unwired: 2 in, 1 out]
                                n467 = local write "D (Rate) IstWert 2"(w1393) -> ()
                                n468 = local write "D (Rate) Sollwert 2"(w1393) -> ()
                                }
                                frame 3 {
                                n469 = String Subset(string=w1398, offset (0)=3) -> (substring=w1399:string)  [unwired: 1 in]
                                n470 = Hexadecimal String To Number(string=w1399) -> (number=w1397:u32)  [unwired: 2 in, 1 out]
                                n471 = local write "% LOW Istwert 2"(w1397) -> ()
                                n472 = local write "% LOW Sollwert 2"(w1397) -> ()
                                }
                                frame 4 {
                                n473 = String Subset(string=w1402, offset (0)=3) -> (substring=w1403:string)  [unwired: 1 in]
                                n474 = Hexadecimal String To Number(string=w1403) -> (number=w1401:u32)  [unwired: 2 in, 1 out]
                                n475 = local write "% HIGH Istwert 2"(w1401) -> ()
                                n476 = local write "% High Sollwert 2"(w1401) -> ()
                                }
                                frame 5 {
                                n477 = call "I3252_Edit_Setpoint.vi"("Read String"=w1406) -> ("Setpoint is"=w1405:dbl)
                                n478 = local write "SP 2 is (°C)"(w1405) -> ()
                                }
                              }
                            }
                          }
                        }
                      }
                      frame #2 {
                        n479 = property on="RAM 2" class="Bool (strict)"("Blinking"=FALSE) -> ()  [unwired: 2 in, 2 out]
                      }
                    }
                    n480 = Not(x="RAM 2") -> (.not. x?=w1341:bool)
                    n481 = Unbundle(w1339) -> ("VISA resource name out"=w1338:refnum<visa-resource-name>, "error out"=w1337:errorcluster)  [unwired: 2 out]
                  }
                  event "Set Gauge to Zero": Value Change {
                    n482 = event-data() -> ()  [unwired: 1 in, 1 out]
                    n483 = flat-sequence {
                      tunnel: w1415 -> [w1420]
                      tunnel: [w1420] -> w1414
                      tunnel: w1414 -> [w1422]
                      tunnel: [w1426] -> w1413
                      tunnel: [w1425] -> w1412
                      tunnel: [w1422] -> w1411
                      tunnel: w1413 -> [w1432]
                      tunnel: w1412 -> [w1431]
                      tunnel: w1411 -> [w1427]
                      frame #0 {
                        n484 = property on="Set Gauge to Zero" class="Bool"("Blinking"=TRUE) -> ()  [unwired: 2 in, 2 out]
                      }
                      frame #1 {
                        w1423 = 0 items=["sensor 1", "sensor 2", "test"] ("Sensor Nr.:")
                        n485 = call "DUAL GAUGE-Get Pressure,Status.vi"("Sensor Nr.:"=w1423, "Referenz in"=w1422) -> ("Pressure"=w1426:dbl)  [unwired: 6 in, 3 out]
                        n486 = call "DUAL GAUGE-Offset display.vi"("W/R"=FALSE, "Referenz in"=w1422) -> ("Sensor 1 Get"=w1425:dbl)  [unwired: 6 in, 3 out]
                      }
                      frame #2 {
                        n487 = Add(x=w1432, y=w1431) -> (x+y=w1428:dbl)
                        n488 = call "DUAL GAUGE-Offset display.vi"("W/R"=TRUE, "Sensor 1 Set"=w1428, "Referenz in"=w1427) -> ("Sensor 1 Get"=→"Current Offset (mbar)":dbl)  [unwired: 5 in, 3 out]
                      }
                      frame #3 {
                        n489 = property on="Set Gauge to Zero" class="Bool"("Blinking"=TRUE) -> ()  [unwired: 2 in, 2 out]
                      }
                    }
                    n490 = Unbundle(w1419) -> ("VISA resource name out"=w1418:refnum<visa-resource-name>, "error out"=w1417:errorcluster)  [unwired: 2 out]
                    n491 = Unbundle(w1410) -> ("VISA resource name out"=w1409:refnum<visa-resource-name>, "error out"=w1408:errorcluster)  [unwired: 2 out]
                  }
                  event "Write to File": Value Change {
                    n492 = event-data() -> ("NewVal"=w1441:bool)  [unwired: 1 in]
                    n493 = Unbundle(w1444) -> ("VISA resource name out"=w1443:refnum<visa-resource-name>, "error out"=w1442:errorcluster)  [unwired: 2 out]
                    n494 = local read "File Path"() -> (w1437:path)
                    n495 = case shown="True" w1441 {
                      tunnel: w1437 -> [_ w1449]
                      tunnel: "User" -> [_ w1448]
                      tunnel: "Sample" -> [_ w1447]
                      tunnel: [path "" ("File Path") w1446] -> w1438
                      frame False {
                      }
                      frame True {
                        n496 = call "Header.vi"("Sample"=w1447, "User"=w1448, "File Path"=w1449) -> ("File Path"=w1446:path)
                      }
                    }
                    n497 = local write "File Path"(w1438) -> ()
                    n498 = Unbundle(w1436) -> ("VISA resource name out"=w1435:refnum<visa-resource-name>, "error out"=w1434:errorcluster)  [unwired: 2 out]
                  }
                }
              }
              n499 = Bundle(cluster=w419, "VISA resource name out"=w418, "error out"=w417) -> (w416:T7)  [unwired: 2 in]
              n500 = Bundle(cluster=w395, "VISA resource name out"=w397, "error out"=w396) -> (w394:T8)  [unwired: 2 in]
            }
            frame #2 {
            }
            frame #3 {
              (unwired) "Daniel Schuster (geb. 20.03.1988)"
              n501 = node-c288(w1512) -> (w1521:T3)  [unwired: 2 in]
              n502 = node-c288(w1527) -> (w1530:T3)  [unwired: 2 in]
              n503 = node-c288(w1517) -> (w1519:T3)  [unwired: 2 in]
              n504 = node-c288(w1526) -> (w1534:T3)  [unwired: 2 in]
              n505 = timed-sequence {
                timing: w1521 -> [_]
                timing-out: [_] -> w1520
                tunnel: w1496 -> [w1608]
                tunnel: w1495 -> [w1604]
                tunnel: [w1607] -> w1488
                tunnel: w1487 -> [w1606]
                tunnel: w1486 -> [w1605]
                tunnel: [w1603] -> w1485
                tunnel: [w1602] -> w1484
                tunnel: [w1601] -> w1482
                n506 = timed-flat-sequence {
                  tunnel: w1608 -> [w1617]
                  tunnel: [w1616] -> w1607
                  tunnel: w1606 -> [w1615]
                  tunnel: w1605 -> [w1614]
                  tunnel: w1604 -> [w1613]
                  tunnel: [w1611] -> w1603
                  tunnel: [w1610] -> w1602
                  tunnel: [w1609] -> w1601
                  n507 = node-c288() -> ()  [unwired: 1 in, 1 out]
                  n508 = case shown="True" "ON (TPG 2)" {
                    tunnel: w1613 -> [w1622 w1628]
                    tunnel: w1614 -> [w1621 w1627]
                    tunnel: [w1620 w1626] -> w1610
                    tunnel: [w1619 w1625] -> w1609
                    frame False {
                      w1623 = 0.0 ("Pressure")
                      n509 = property on="ON (TPG 2)" class="Bool (strict)"("Blinking"=FALSE) -> ()  [unwired: 2 in, 2 out]
                      n510 = Bundle("Pressure"=w1623, "Pressure"=w1623) -> (w1620:cluster{"Pressure":dbl, "Pressure":dbl})  [unwired: 1 in]
                      n511 = Bundle("TPG 2 COM"=w1622, "error out"=w1621) -> (w1619:T9)  [unwired: 1 in]
                    }
                    frame True {
                      n512 = stacked-sequence {
                        tunnel: w1628 -> [_ w1641]
                        tunnel: [_ w1637] -> w1626
                        tunnel: [_ w1633] -> w1625
                        tunnel: w1627 -> [_ w1630]
                        frame #0 {
                          n513 = property on="ON (TPG 2)" class="Bool (strict)"("Blinking"=TRUE) -> ()  [unwired: 2 in, 2 out]
                        }
                        frame #1 {
                          n514 = call "PresureGetSubVI.vi"("COM in"=w1641, "Fehler (Eingang)"=w1630) -> ("Status Gauge#1"=→"Status Gauge 2#1":i32, "Status Gauge#2"=→"Status Gauge 2#2":i32, "COM out"=w1634:refnum<visa-resource-name>, "Pressure Gauge#1"=w1635:dbl, "Pressure Gauge#2"=w1638:dbl, "Cluster (Ausgang)"=w1631:errorcluster)  [unwired: 12 in]
                          "Pressure Gauge 2#1" <- w1635
                          "Pressure Gauge 2#2" <- w1638
                          n515 = Bundle("COM out"=w1634, "Cluster (Ausgang)"=w1631) -> (w1633:T10)  [unwired: 1 in]
                          n516 = Unbundle(w1631) -> ("status"=w1632:bool, "code"=w1636:i32)  [unwired: 1 out]
                          n517 = Bundle("status"=w1632, "code"=w1636) -> ()  [unwired: 1 in, 1 out]
                          n518 = Bundle("Pressure Gauge#1"=w1635, "Pressure Gauge#2"=w1638) -> (w1637:T11)  [unwired: 1 in]
                        }
                      }
                    }
                  }
                  n519 = case shown="True" "ON (TPG 1)" {
                    tunnel: w1617 -> [w1645 w1651]
                    tunnel: [w1644 w1650] -> w1616
                    tunnel: w1615 -> [w1643 w1649]
                    tunnel: [w1642 w1648] -> w1611
                    frame False {
                      w1646 = 0.0 ("Pressure")
                      n520 = property on="ON (TPG 1)" class="Bool (strict)"("Blinking"=FALSE) -> ()  [unwired: 2 in, 2 out]
                      n521 = Bundle("Pressure"=w1646, "Pressure"=w1646) -> (w1642:cluster{"Pressure":dbl, "Pressure":dbl})  [unwired: 1 in]
                      n522 = Bundle("TPG 1 COM"=w1645, "error out"=w1643) -> (w1644:T12)  [unwired: 1 in]
                    }
                    frame True {
                      n523 = stacked-sequence {
                        tunnel: w1651 -> [_ w1664]
                        tunnel: [_ w1657] -> w1650
                        tunnel: w1649 -> [_ w1654]
                        tunnel: [_ w1653] -> w1648
                        frame #0 {
                          n524 = property on="ON (TPG 1)" class="Bool (strict)"("Blinking"=TRUE) -> ()  [unwired: 2 in, 2 out]
                        }
                        frame #1 {
                          n525 = call "PresureGetSubVI.vi"("COM in"=w1664, "Fehler (Eingang)"=w1654) -> ("Status Gauge#1"=→"Status Gauge 1#1":i32, "Status Gauge#2"=→"Status Gauge 1#2":i32, "COM out"=w1658:refnum<visa-resource-name>, "Pressure Gauge#1"=w1659:dbl, "Pressure Gauge#2"=w1661:dbl, "Cluster (Ausgang)"=w1655:errorcluster)  [unwired: 12 in]
                          "Pressure Gauge 1#1" <- w1659
                          "Pressure Gauge 1#2" <- w1661
                          n526 = Bundle("COM out"=w1658, "Cluster (Ausgang)"=w1655) -> (w1657:T10)  [unwired: 1 in]
                          n527 = Unbundle(w1655) -> ("status"=w1656:bool, "code"=w1660:i32)  [unwired: 1 out]
                          n528 = Bundle("status"=w1656, "code"=w1660) -> ()  [unwired: 1 in, 1 out]
                          n529 = Bundle("Pressure Gauge#1"=w1659, "Pressure Gauge#2"=w1661) -> (w1653:T11)  [unwired: 1 in]
                        }
                      }
                    }
                  }
                  n530 = node-c288() -> ()  [unwired: 1 in, 1 out]
                }
              }
              n531 = timed-sequence {
                timing: w1530 -> [_]
                timing-out: [_] -> w1529
                tunnel: w1528 -> [w1674]
                tunnel: [w1673] -> w1523
                tunnel: [w1672] -> w1522
                tunnel: [w1671] -> w1509
                n532 = timed-flat-sequence {
                  tunnel: w1674 -> [w1678]
                  tunnel: [w1677] -> w1673
                  tunnel: [w1676] -> w1672
                  tunnel: [w1675] -> w1671
                  n533 = node-c288() -> ()  [unwired: 1 in, 1 out]
                  n534 = case shown="True" "ON" {
                    tunnel: w1678 -> [w1682 w1687]
                    tunnel: [w1681 w1686] -> w1677
                    tunnel: [w1680 w1685] -> w1676
                    tunnel: [_ w1684] -> w1675
                    frame False {
                      n535 = Unbundle(w1682) -> ("VISA resource name out"=w1681:refnum<visa-resource-name>, "error out"=w1680:errorcluster)  [unwired: 2 out]
                      n536 = property on="ON" class="Bool (strict)"("Blinking"=FALSE) -> ()  [unwired: 2 in, 2 out]
                    }
                    frame True {
                      n537 = stacked-sequence {
                        tunnel: w1687 -> [_ w1692]
                        tunnel: [_ w1691] -> w1686
                        tunnel: [_ w1690] -> w1685
                        tunnel: [_ w1689] -> w1684
                        frame #0 {
                          n538 = property on="ON" class="Bool (strict)"("Blinking"=TRUE) -> ()  [unwired: 2 in, 2 out]
                        }
                        frame #1 {
                          n539 = Unbundle(w1692) -> ("VISA resource name out"=w1696:refnum<visa-resource-name>, "error out"=w1694:errorcluster, "Delay (ms)"=w1695:u32, "Write/\nRead"=w1693:bool)
                          n540 = call "I3252_Comm_Interface.vi"("VISA resource name in"=w1696, "error in"=w1694, "Delay (ms)"=w1695, "Write"=w1693, "String to Write"="*V01", "Read"=w1693) -> ("VISA resource name out"=w1691:refnum<visa-resource-name>, "error out"=w1690:errorcluster, "Read String"=w1689:string)  [unwired: 2 in]
                        }
                      }
                    }
                  }
                  n541 = node-c288() -> ()  [unwired: 1 in, 1 out]
                }
              }
              n542 = timed-sequence {
                timing: w1519 -> [_]
                timing-out: [_] -> w1518
                tunnel: w1516 -> [w1570]
                tunnel: w1515 -> [w1569]
                tunnel: [w1568] -> w1513
                tunnel: [w1567] -> w1514
                tunnel: [w1566] -> w1510
                n543 = timed-flat-sequence {
                  tunnel: w1570 -> [w1575]
                  tunnel: w1569 -> [w1574]
                  tunnel: [w1573] -> w1568
                  tunnel: [w1572] -> w1567
                  tunnel: [w1571] -> w1566
                  n544 = node-c288() -> ()  [unwired: 1 in, 1 out]
                  n545 = case shown="False" "ON" {
                    tunnel: w1575 -> [w1579 w1585]
                    tunnel: w1574 -> [w1580 w1584]
                    tunnel: [w1579 w1583] -> w1573
                    tunnel: [w1580 w1582] -> w1572
                    tunnel: [0.0 ("Reading") w1581] -> w1571
                    frame False {
                      n546 = property on="ON" class="Bool (strict)"("Blinking"=FALSE) -> ()  [unwired: 2 in, 2 out]
                    }
                    frame True {
                      n547 = stacked-sequence {
                        tunnel: w1585 -> [_ w1592]
                        tunnel: w1584 -> [_ w1591]
                        tunnel: [_ w1590] -> w1583
                        tunnel: [_ w1589] -> w1582
                        tunnel: [_ w1587] -> w1581
                        frame #0 {
                          n548 = property on="ON" class="Bool (strict)"("Blinking"=TRUE) -> ()  [unwired: 2 in, 2 out]
                        }
                        frame #1 {
                          n549 = call "VC840_Read.vi"("error in (no error)"=w1591, "VISA resource name"=w1592) -> ("error out"=w1589:errorcluster, "Unit"=→"Unit 2":string, "Reading"=w1587:dbl, "VISA resource name out"=w1590:refnum<visa-resource-name>, "Status"=→"Status 2":T2, "Mode"=→"Mode 2":enum16{"?", "Diode", "Beep", "DC", "AC"})  [unwired: 4 out]
                          "Reading 2" <- w1587
                        }
                      }
                    }
                  }
                  n550 = node-c288() -> ()  [unwired: 1 in, 1 out]
                }
              }
              n551 = timed-sequence {
                timing: w1534 -> [_]
                timing-out: [_] -> w1533
                tunnel: w1532 -> [w1708]
                tunnel: w1531 -> [w1707]
                tunnel: [w1706] -> w1525
                tunnel: [w1705] -> w1524
                tunnel: [w1704] -> w1511
                n552 = timed-flat-sequence {
                  tunnel: w1708 -> [w1713]
                  tunnel: w1707 -> [w1712]
                  tunnel: [w1711] -> w1706
                  tunnel: [w1710] -> w1705
                  tunnel: [w1709] -> w1704
                  n553 = node-c288() -> ()  [unwired: 1 in, 1 out]
                  n554 = case shown="False" "ON" {
                    tunnel: w1713 -> [w1717 w1723]
                    tunnel: w1712 -> [w1718 w1722]
                    tunnel: [w1717 w1721] -> w1711
                    tunnel: [w1718 w1720] -> w1710
                    tunnel: [0.0 ("Reading") w1719] -> w1709
                    frame False {
                      n555 = property on="ON" class="Bool (strict)"("Blinking"=FALSE) -> ()  [unwired: 2 in, 2 out]
                    }
                    frame True {
                      n556 = stacked-sequence {
                        tunnel: w1723 -> [_ w1730]
                        tunnel: w1722 -> [_ w1729]
                        tunnel: [_ w1728] -> w1721
                        tunnel: [_ w1727] -> w1720
                        tunnel: [_ w1725] -> w1719
                        frame #0 {
                          n557 = property on="ON" class="Bool (strict)"("Blinking"=TRUE) -> ()  [unwired: 2 in, 2 out]
                        }
                        frame #1 {
                          n558 = call "VC840_Read.vi"("error in (no error)"=w1729, "VISA resource name"=w1730) -> ("error out"=w1727:errorcluster, "Unit"=→"Unit 1":string, "Reading"=w1725:dbl, "VISA resource name out"=w1728:refnum<visa-resource-name>, "Status"=→"Status 1":T2, "Mode"=→"Mode 1":enum16{"?", "Diode", "Beep", "DC", "AC"})  [unwired: 4 out]
                          "Reading 1" <- w1725
                        }
                      }
                    }
                  }
                  n559 = node-c288() -> ()  [unwired: 1 in, 1 out]
                }
              }
              n560 = Tick Count (ms)() -> (millisecond timer value=w1497:u32)
              n561 = Subtract(x=w1497, y=w1502) -> (x-y=w1501:u32)
              n562 = Divide(x=w1501, y=u32 1000) -> (x/y=w1499:dbl)
              n563 = node-c288(w1529) -> ()  [unwired: 1 out]
              n564 = node-c288(w1533) -> ()  [unwired: 1 out]
              n565 = node-c288(w1518) -> ()  [unwired: 1 out]
              n566 = node-c288(w1473) -> (w1480:T3)  [unwired: 2 in]
              n567 = To Double Precision Float(number=w1499) -> (double precision float=w1503:dbl)
              "current time (s)" <- w1503
              n568 = timed-sequence {
                timing: w1480 -> [_]
                timing-out: [_] -> w1479
                tunnel: w1478 -> [w1538]
                tunnel: [w1537] -> w1475
                tunnel: [w1536] -> w1474
                tunnel: [w1535] -> w1477
                n569 = timed-flat-sequence {
                  tunnel: w1538 -> [w1543]
                  tunnel: [w1542] -> w1537
                  tunnel: [w1541] -> w1536
                  tunnel: [w1540] -> w1535
                  n570 = node-c288() -> ()  [unwired: 1 in, 1 out]
                  n571 = case shown="True" "ON 2" {
                    tunnel: w1543 -> [w1546 w1550]
                    tunnel: [w1545 w1549] -> w1542
                    tunnel: [w1544 w1548] -> w1541
                    tunnel: [_ w1547] -> w1540
                    frame False {
                      (unwired) FALSE
                      n572 = Unbundle(w1546) -> ("VISA resource name out"=w1545:refnum<visa-resource-name>, "error out"=w1544:errorcluster)  [unwired: 2 out]
                    }
                    frame True {
                      n573 = stacked-sequence {
                        tunnel: w1550 -> [_ w1554]
                        tunnel: [_ w1553] -> w1549
                        tunnel: [_ w1552] -> w1548
                        tunnel: [_ w1551] -> w1547
                        frame #0 {
                          (unwired) TRUE
                        }
                        frame #1 {
                          n574 = Unbundle(w1554) -> ("VISA resource name out"=w1558:refnum<visa-resource-name>, "error out"=w1556:errorcluster, "Delay (ms) 2"=w1557:u32, "Write/\nRead \n\n2"=w1555:bool)
                          n575 = call "I3252_Comm_Interface.vi"("VISA resource name in"=w1558, "error in"=w1556, "Delay (ms)"=w1557, "Write"=w1555, "String to Write"="*V01", "Read"=w1555) -> ("VISA resource name out"=w1553:refnum<visa-resource-name>, "error out"=w1552:errorcluster, "Read String"=w1551:string)  [unwired: 2 in]
                        }
                      }
                    }
                  }
                  n576 = node-c288() -> ()  [unwired: 1 in, 1 out]
                }
              }
              n577 = node-c288(w1520) -> ()  [unwired: 1 out]
              n578 = Unbundle(w1484) -> ("Pressure Gauge#1"=w1483:dbl, "Pressure Gauge#2"=w1481:dbl)
              "Pressure OpenPort2" <- w1481
              "Pressure Pirani 2" <- w1483
              n579 = Unbundle(w1485) -> ("Pressure Gauge#1"=w1494:dbl, "Pressure Gauge#2"=w1489:dbl)
              "Pressure Baratron 2" <- w1494
              "Pressure FullRange 2" <- w1489
              n580 = node-c288(w1479) -> ()  [unwired: 1 out]
            }
            frame #4 {
              n581 = Build Array (concatenate)(w1756, w1760) -> (w1755:dbl[])
              n582 = Build Array (concatenate)(w1759, w1761) -> (w1754:dbl[])
              n583 = Build Array (concatenate)(w1757, w1748) -> (w1752:dbl[])
              n584 = Build Array (concatenate)(w1758, w1749) -> (w1753:dbl[])
              n585 = Greater?(x=w1780, y="Pressure Limit (mbar)") -> (0:w1783:bool)
              n586 = case shown="False" w1783 {
                frame False {
                  w1793 = T6."Enabled" ("Disabled")
                  n587 = property on="Standby" class="Bool (strict)"("DisabledEnum"=w1793) -> ()  [unwired: 2 in, 2 out]
                  n588 = property on="Standby\n2" class="Bool (strict)"("DisabledEnum"=w1793) -> ()  [unwired: 2 in, 2 out]
                }
                frame True {
                  w1795 = T6."Disabled" ("Disabled")
                  w1794 = TRUE ("Standby")
                  n589 = property on="Standby" class="Bool (strict)"("Val(Sgnl)"=w1794, "DisabledEnum"=w1795) -> ()  [unwired: 2 in, 2 out]
                  n590 = property on="Standby\n2" class="Bool (strict)"("Val(Sgnl)"=w1794, "DisabledEnum"=w1795) -> ()  [unwired: 2 in, 2 out]
                }
              }
              n591 = call "Resistivity_Calculation.vi"("Reading 1 (V)"=w1773, "Constant"="4PP constant", "Thickness (nm)"="Thickness (nm)", "Reading 2 (A)"=w1781) -> ("Resivtivity (Ohm*cm)"=w1765:dbl, "Current"=w1766:dbl, "Voltage"=w1767:dbl)
              "Resistivity (Ohm*cm)" <- w1765
              "Voltage (V)" <- w1767
              "Current (A)" <- w1766
              n592 = call "I3252_Edit_Temperature.vi"("Temp. String"=w1782) -> ("Temp. (°C)"=w1776:dbl)
              "(°C)" <- w1776
              n593 = call "I3252_Edit_Temperature.vi"("Temp. String"=w1744) -> ("Temp. (°C)"=w1739:dbl)
              "(°C) 2" <- w1739
              n594 = Build Array (concatenate)(w1778, w1779) -> (w1775:dbl[])
              n595 = Build Array (concatenate)(w1777, w1776) -> (w1763:dbl[])
              n596 = Build Array (concatenate)(w1742, w1739) -> (w1743:dbl[])
              n597 = Build Array (concatenate)(w1774, w1767) -> (w1772:dbl[])
              n598 = Build Array (concatenate)(w1771, w1766) -> (w1769:dbl[])
              n599 = Build Array (concatenate)(w1770, w1765) -> (w1768:dbl[])
              n600 = Build Array(w1767, w1766, w1765) -> (w1764:dbl[])
            }
            frame #5 {
              n601 = Bundle(w1807, w1822) -> (→"CMR275 Baratron":cluster{dbl[], dbl[]})  [unwired: 1 in]
              n602 = Bundle(w1807, w1821) -> (w1801:cluster{dbl[], dbl[]})  [unwired: 1 in]
              n603 = Bundle(w1807, w1820) -> (w1800:cluster{dbl[], dbl[]})  [unwired: 1 in]
              n604 = Bundle(w1807, w1819) -> (→"Pressure OpenPort":cluster{dbl[], dbl[]})  [unwired: 1 in]
              n605 = Bundle(w1807, w1826) -> (w1803:cluster{dbl[], dbl[]})  [unwired: 1 in]
              n606 = Bundle(w1807, w1827) -> (→"Voltage":cluster{dbl[], dbl[]})  [unwired: 1 in]
              n607 = Bundle(w1807, w1828) -> (→"Current":cluster{dbl[], dbl[]})  [unwired: 1 in]
              n608 = Bundle(w1807, w1829) -> (→"Resistivity":cluster{dbl[], dbl[]})  [unwired: 1 in]
              n609 = Bundle(w1807, w1808) -> (w1804:cluster{dbl[], dbl[]})  [unwired: 1 in]
              n610 = Build Array(w1801, w1800) -> (→"Pirani (VVP1 Scroll)":cluster{dbl[], dbl[]}[])
              n611 = Build Array(w1803, w1804) -> (→"TEMPERATURE":cluster{dbl[], dbl[]}[])
              n612 = Build Array (concatenate)(w1798, w1797, w1796, w1833, w1825, w1814, w1811, w1809) -> (w1840:dbl[])
              "appended array" <- w1840
            }
            frame #6 {
              n613 = Unbundle(w1853) -> ("COM out"=w1852:refnum<visa-resource-name>, "Cluster (Ausgang)"=w1851:errorcluster)
              n614 = Unbundle(w1850) -> ("COM out"=w1849:refnum<visa-resource-name>, "Cluster (Ausgang)"=w1848:errorcluster)
              n615 = call "Elapsed Time"("Time Target (s)"="Intervall (s)") -> ("Time has Elapsed"=w1842:bool)  [unwired: 11 in, 7 out]
              n616 = And(x="Write to File", y=w1842) -> (x .and. y?=w1841:bool)
              n617 = case shown="False" w1841 {
                tunnel: [w1875 w1881] -> w1867
                tunnel: "File Path" -> [w1875 w1879]
                tunnel: w1860 -> [_ w1877]
                frame False {
                  n618 = property on="Write to File" class="Bool (strict)"("Blinking"=FALSE) -> ()  [unwired: 2 in, 2 out]
                }
                frame True {
                  n619 = flat-sequence {
                    tunnel: [w1883] -> w1880
                    tunnel: w1879 -> [w1883]
                    tunnel: [w1882] -> w1878
                    tunnel: w1877 -> [w1882]
                    tunnel: [w1888] -> w1881
                    tunnel: w1880 -> [w1887]
                    tunnel: w1878 -> [w1886]
                    frame #0 {
                      n620 = property on="Write to File" class="Bool (strict)"("Blinking"=TRUE) -> ()  [unwired: 2 in, 2 out]
                    }
                    frame #1 {
                      n621 = call-poly <vilib>:"Write To Spreadsheet File.vi"("format (%.3f)"="%g", "append to file? (new file:F)"=TRUE ("transpose? (no:F)"), "1D data"=w1886, "file path (dialog if empty)"=w1887) -> ("new file path (Not A Path if cancelled)"=w1888:path)  [unwired: 4 in]
                    }
                  }
                }
              }
              n622 = Merge Errors(w1871, w1870, w1868, w1851, w1848) -> (w1869:errorcluster)
              n623 = call <vilib>:"Simple Error Handler.vi"("error in (no error)"=w1869) -> ("error?"=w1854:bool)  [unwired: 4 in, 4 out]
              n624 = local write "File Path"(w1867) -> ()
            }
            frame #7 {
              w1908 = u32 1000 ("y")
              # "TEMP"
              n625 = Tick Count (ms)() -> (millisecond timer value=w1910:u32)
              n626 = Subtract(x=w1910, y=w1909) -> (x-y=w1911:u32)
              n627 = VISA Flush I/O Buffer(VISA resource name=w1902, error in (no error)=w1901) -> (VISA resource name out=w1899:refnum<visa-resource-name>, error out=w1900:errorcluster)  [unwired: 1 in]
              n628 = VISA Flush I/O Buffer(VISA resource name=w1895, error in (no error)=w1894) -> (VISA resource name out=w1898:refnum<visa-resource-name>, error out=w1897:errorcluster)  [unwired: 1 in]
              n629 = Divide(x=w1911, y=w1908) -> (x/y=→"loop time (s)":dbl)
              n630 = Subtract(x=u32 1, y=u32 1) -> (x-y=w1912:u32)
              n631 = Multiply(x=w1912, y=w1908) -> (x*y=w1914:u32)
              n632 = Wait (ms)(milliseconds to wait=w1914) -> ()  [unwired: 1 out]
              n633 = Bundle("COM out"=w1899, "error out"=w1900, "COM out"=w1898, "error out"=w1897) -> (w1896:T13)  [unwired: 1 in]
            }
            frame #8 {
              n634 = Tick Count (ms)() -> (millisecond timer value=w1937:u32)
              n635 = Subtract(x=w1937, y=w1935) -> (x-y=w1936:u32)
              n636 = Divide(x=w1936, y=w1934) -> (x/y=→"data logger intervall (s)":dbl)
            }
          }
          n637 = Exclusive Or(1:"stop", 2:w176) -> (0:w177:bool)
        }
      }
      frame #4 {
        n638 = call "VC840_Close.vi"("error in (no error)"=w1959, "VISA resource name"=w1960) -> ("error out"=w1968:errorcluster)  [unwired: 9 in]
        n639 = call "VC840_Close.vi"("error in (no error)"=w1961, "VISA resource name"=w1962) -> ("error out"=w1966:errorcluster)  [unwired: 9 in]
        n640 = VISA Close(VISA resource name=w1964, error in (no error)=w1963) -> (error out=w1965:errorcluster)
        n641 = VISA Close(VISA resource name=w1952, error in (no error)=w1951) -> (error out=w1950:errorcluster)
        n642 = Unbundle(w1957) -> ("COM out"=w1956:refnum<visa-resource-name>, "error out"=w1955:errorcluster, "COM out"=w1953:refnum<visa-resource-name>, "error out"=w1954:errorcluster)
        n643 = VISA Close(VISA resource name=w1956, error in (no error)=w1955) -> ()  [unwired: 1 out]
        n644 = VISA Close(VISA resource name=w1953, error in (no error)=w1954) -> ()  [unwired: 1 out]
        n645 = Merge Errors(w1965, w1966, w1968, w1950) -> (w1967:errorcluster)
        n646 = call <vilib>:"Simple Error Handler.vi"("error in (no error)"=w1967) -> ("error?"=w1958:bool)  [unwired: 1 in, 7 out]
        n647 = Stop(stop? (T)=w1958) -> ()
      }
    }
  }
